vi "多道分析仪.vi"() -> ()   [LabVIEW 2014]
uses:
  <vilib>/Utility/miscctls.llb/LVPointDoubleTypeDef.ctl
  <vilib>/Utility/file.llb/Read From Spreadsheet File (DBL).vi
  <vilib>/Utility/file.llb/Write To Spreadsheet File (DBL).vi
  <vilib>/Analysis/NI_AAL_SigProc.lvlib
  <vilib>/Analysis/NI_AALPro.lvlib
panel:
  in  "按钮_对数":bool caption="对数"
  out "变量：显示数据":dbl[](array[numeric])
  out "状态：本次测量和上次未完成测量时间和":dbl
  out "状态：本次测试已测时间":dbl
  out "状态：上次未完成测试的已测时间":dbl
  out "变量：每次测量计划用时":u16=3600
  out "设置：幅度谱总道数 2":u32=4096
  out "变量：实时计数":i32
  out "变量：剩余使用时间":dbl
  out "center":dbl caption="中心"
  in  "设置：信号极性（正T）":bool=TRUE
  in  "数据缓存索引":u32
  out "变量 : 实时总计数":u64
  out "设置 ： 修正文件路径":path
  out "变量 ： 上次测量总计数":u32
  out "变量：上次测量原始数据":dbl[](array[numeric])
  out "状态：已测时间":dbl
  out "状态：测量开始时间":u32
  out "状态：刷新次数":i32
  in  "状态：停止变量":bool=TRUE
  out "变量：上次测量时间":dbl
  out "变量：原始数据":dbl[](array[numeric])
  out "MCA道宽修正数组":ext[](array[numeric])
  in  "设置：寻峰灵敏度":i32=3 caption="宽度" min=3
  in  "设置：甄别前阈值":u16=10000
  in  "设置：甄别后阈值":u16=9000
  in  "设置：刷新频率":u16
  in  "设置：测量时间":u16
  out "结果：净面积":dbl=1313865.0
  out "结果：半高宽":dbl=218.0
  out "结果：峰位":dbl=1585.0 caption="中心"
  in  "按钮_游标":bool caption="游标"
  in  "按钮_寻峰":T1 caption="寻峰"
  in  "按钮_右移":bool caption="右移"
  in  "按钮_还原":bool caption="还原"
  in  "按钮_放大":bool caption="放大"
  in  "按钮_左移":bool caption="左移"
  out "变量：感兴区终点道址":dbl=-1.0
  in  "显示：列表显示内容":string[](array[string])=["", "0秒", "正", "9000", "10000", "", "", "2014年3月7日", "0:56:44", "0秒", "0", "", "", "", "", "", "", "", "", "", "", ""]
  out "变量：感兴区起点道址":dbl=-1.0
  out "设置：幅度谱总道数":u32=4096
  in  "变量：图像缓存数组":dbl[][](array[numeric])
  in  "按钮_退出":bool caption="退出"
  in  "按钮_帮助":bool caption="帮助"
  in  "按钮_复位":bool caption="复位"
  in  "按钮_停止":bool caption="停止"
  in  "按钮_开始":bool caption="开始"
  in  "按钮_设置":bool caption="设置"
  in  "按钮_保存":bool caption="保存"
  in  "按钮_打开":bool caption="打开"
  out "显示：波形图":dbl[][](graph)
  out "显示：列表框":T2=6
  out "显示：波形图_预览":dbl[][](graph)
  out "状态栏_仪器状态":T3="核电子学硬件平台未连接" caption="状态栏"
  out "状态栏_剩余使用时间":T3="0" caption="剩余使用时间："
  out "状态栏_计数率":T3="0" caption="实时计数率："
  out "状态栏_游标状态":T3="隐藏" caption="游标状态："
  out "状态栏_游标计数":T3="0" caption="游标计数："
  out "状态栏_游标道址":T3="0" caption="游标道址："
  out "状态栏_测量状态":T3="停止" caption="测量状态："
  out "状态栏_日期":T3="2014/3/7   0:56:56" caption="日期"
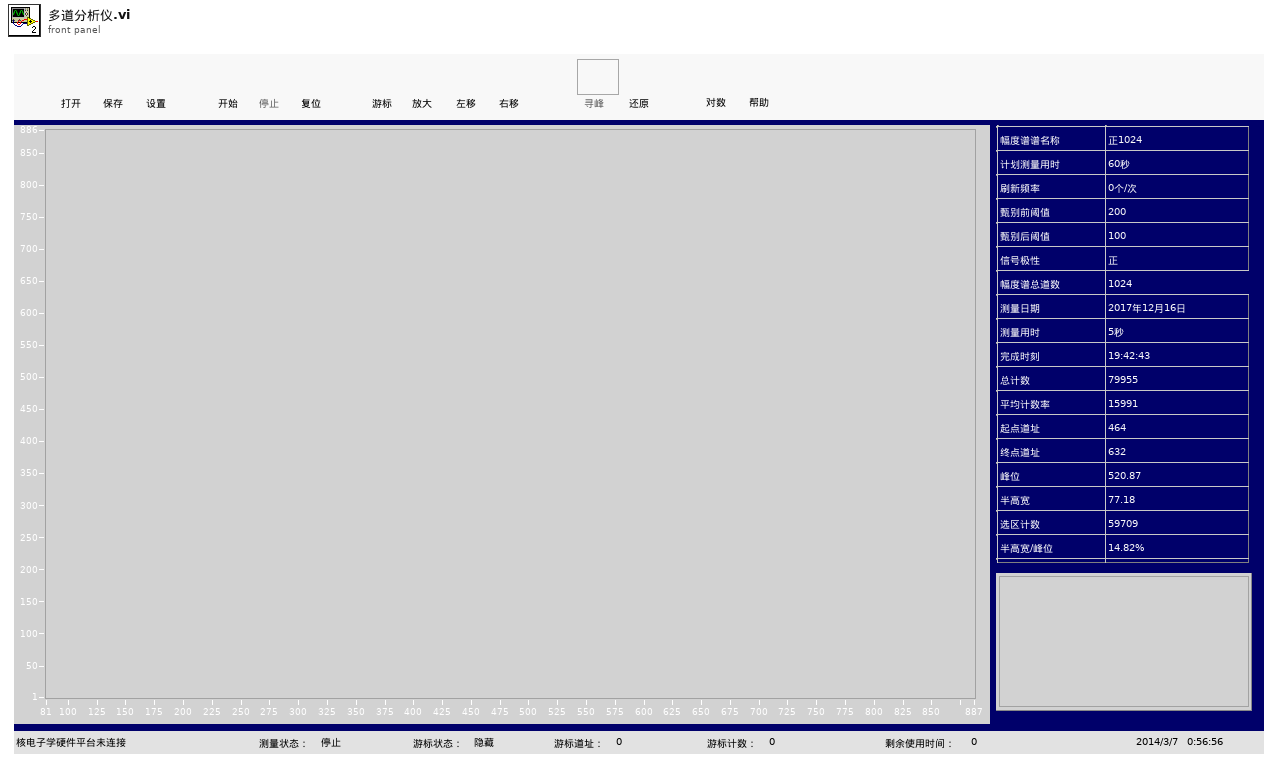
[diagram p1: front panel]
types:
  T1 = typedef "寻峰控件.ctl" = bool
  T2 = typedef "透明表格.ctl" = i32
  T3 = typedef "透明字符串.ctl" = string
  T4 = typedef "枚举常量_状态机.ctl" = enum16{"初始化", "等待", "完成"}
  T5 = typedef "LVPointDoubleTypeDef.ctl" = cluster{"X":dbl, "Y":dbl}
  T6 = enum8{"Enabled", "Disabled", "Disabled and Grayed Out"}
  T7 = enum16{"open", "open or create", "create or replace", "create", "open (read-only)"}
  T8 = typedef "eventvkey.ctl" = enum16{"ASCII", "Enter", "Return", "Shift", "Ctrl", "Alt", "Cmd", "Opt", "Caps", "NumLock", "Clear", "Break", "Up", "Down", "Left", "Right", "Insert", "Delete", "Home", "End", "PageUp", "PageDown", "Escape", "Help", "Pause", "ScrollLock", "F1", "F2", "F3", "F4", "F5", "F6", "F7", "F8", "F9", "F10", "F11", "F12", "F13", "F14", "F15", "F16", "F17", "F18", "F19", "F20", "F21", "F22", "F23", "F24", "Play", "VolumeUp", "VolumeDown", "Mute", "Two Byte Char"}
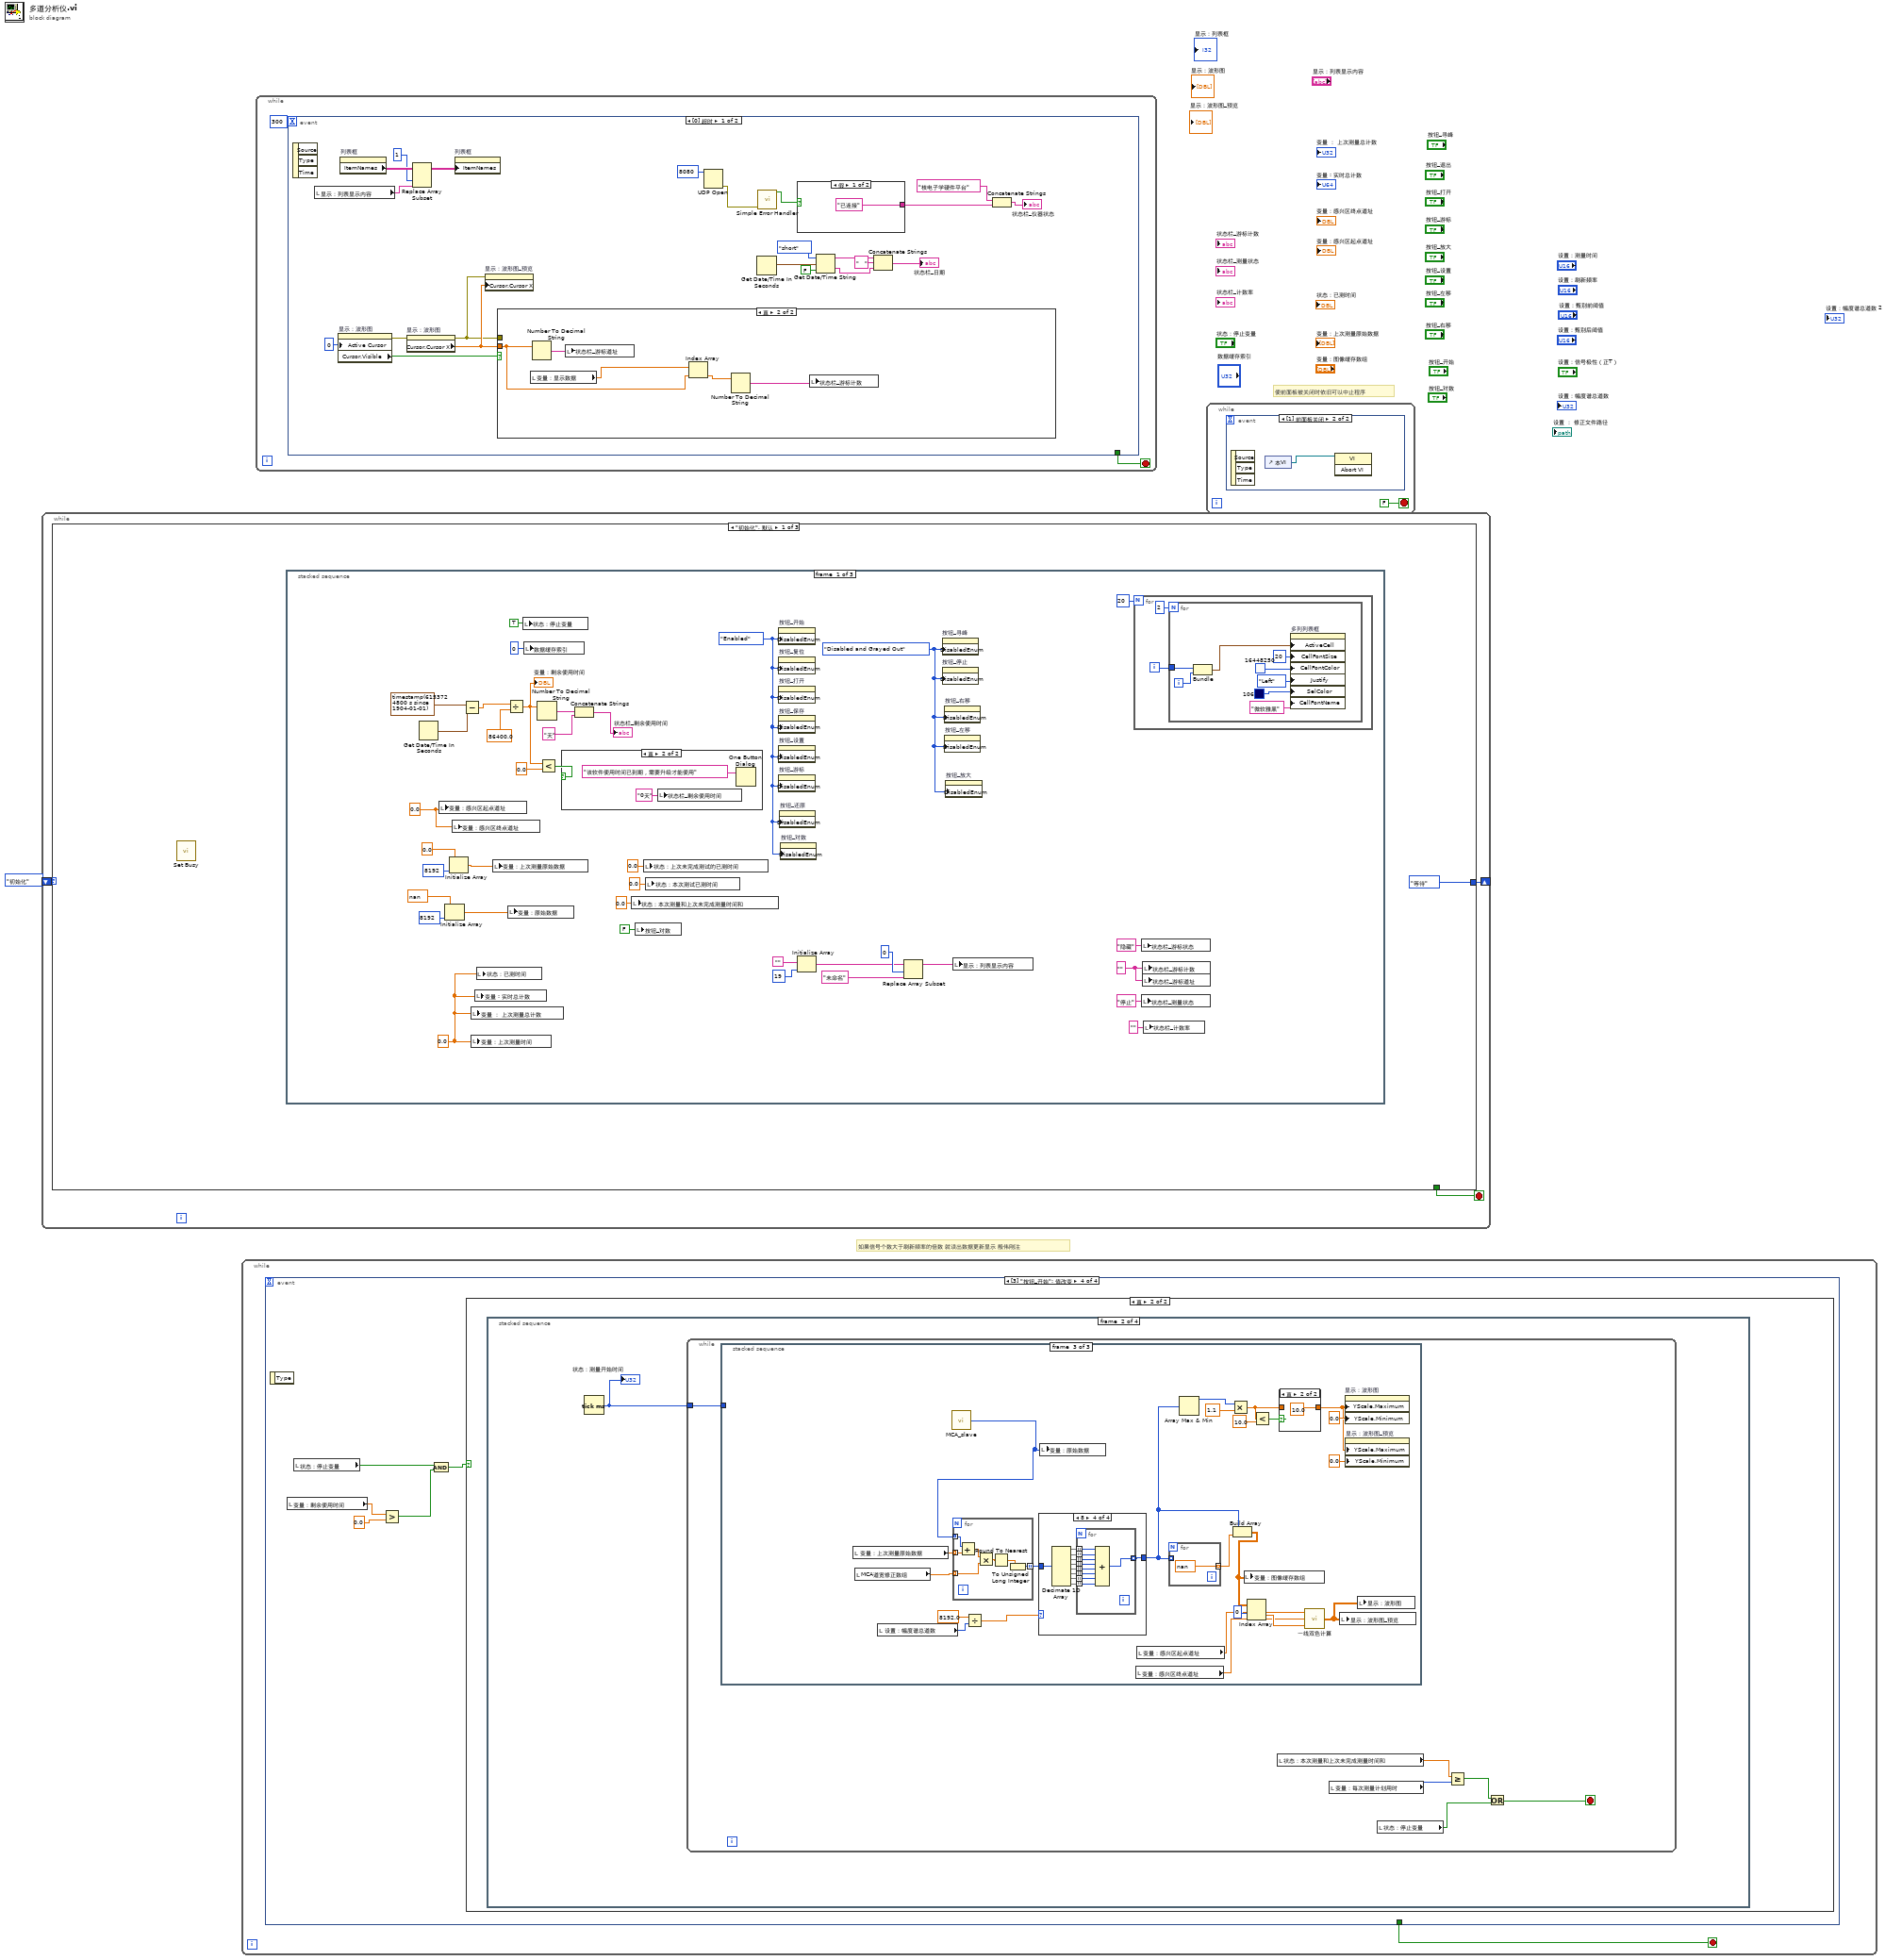
[diagram p0: block diagram]
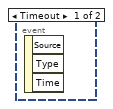
[diagram p2: hidden frame]
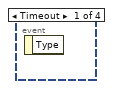
[diagram p3: hidden frame]
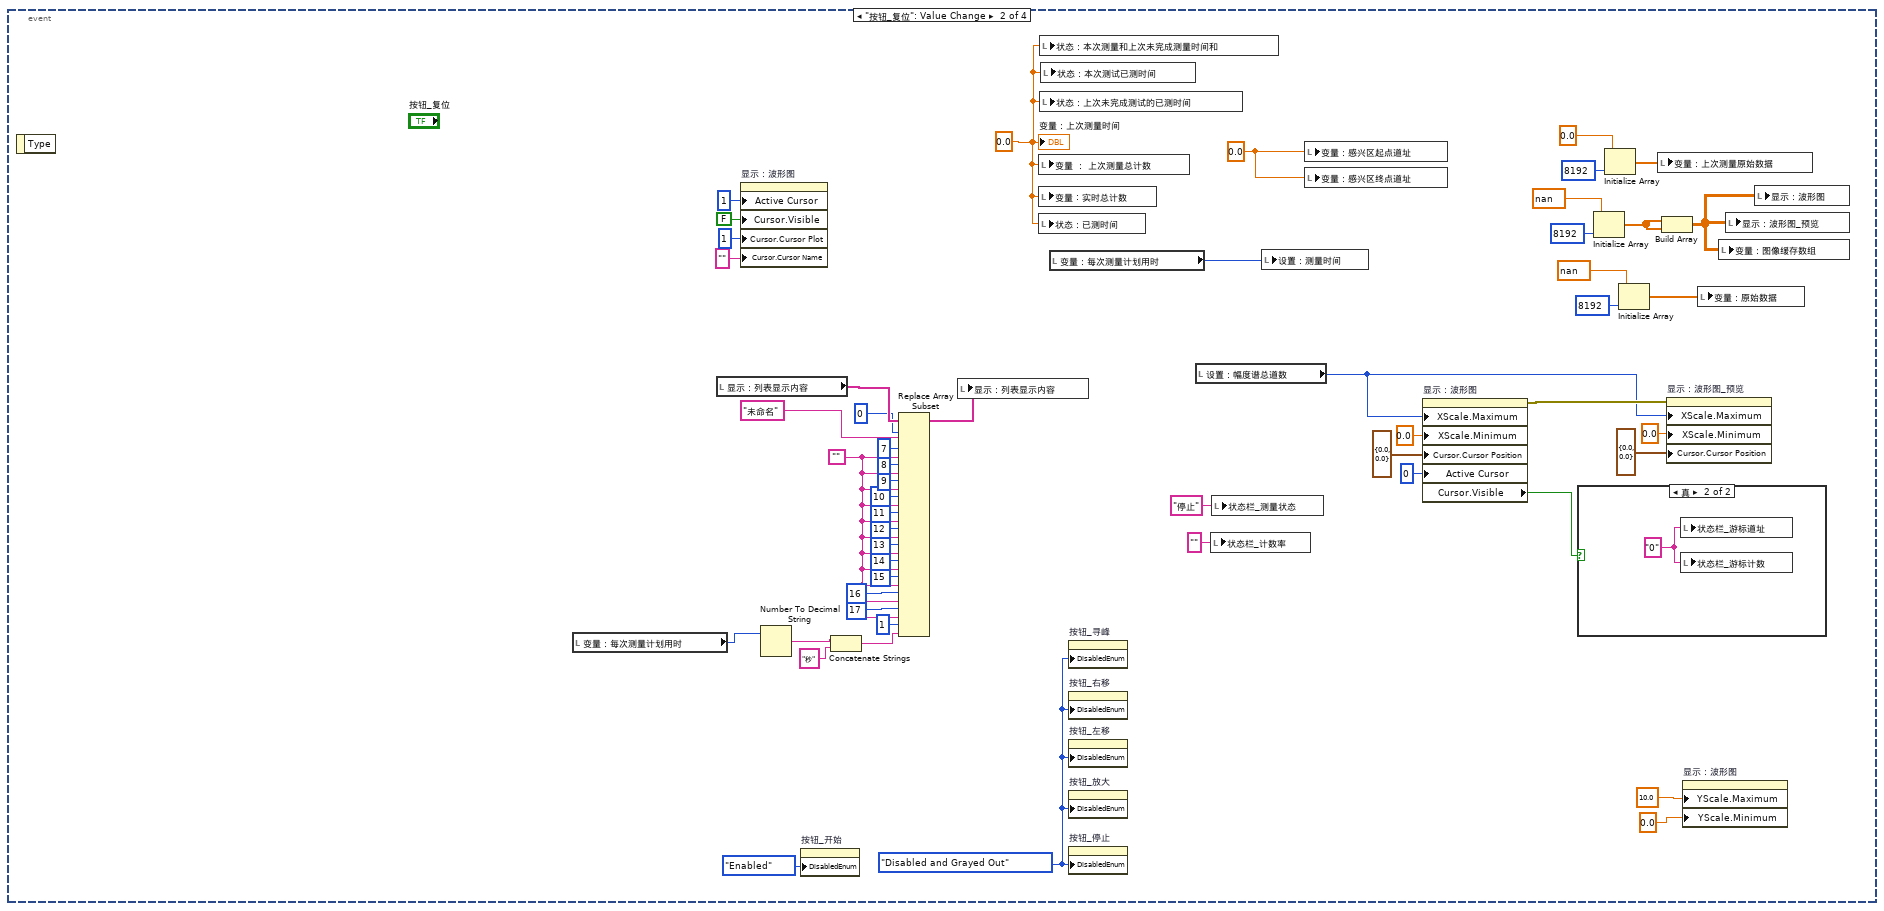
[diagram p4: hidden frame]
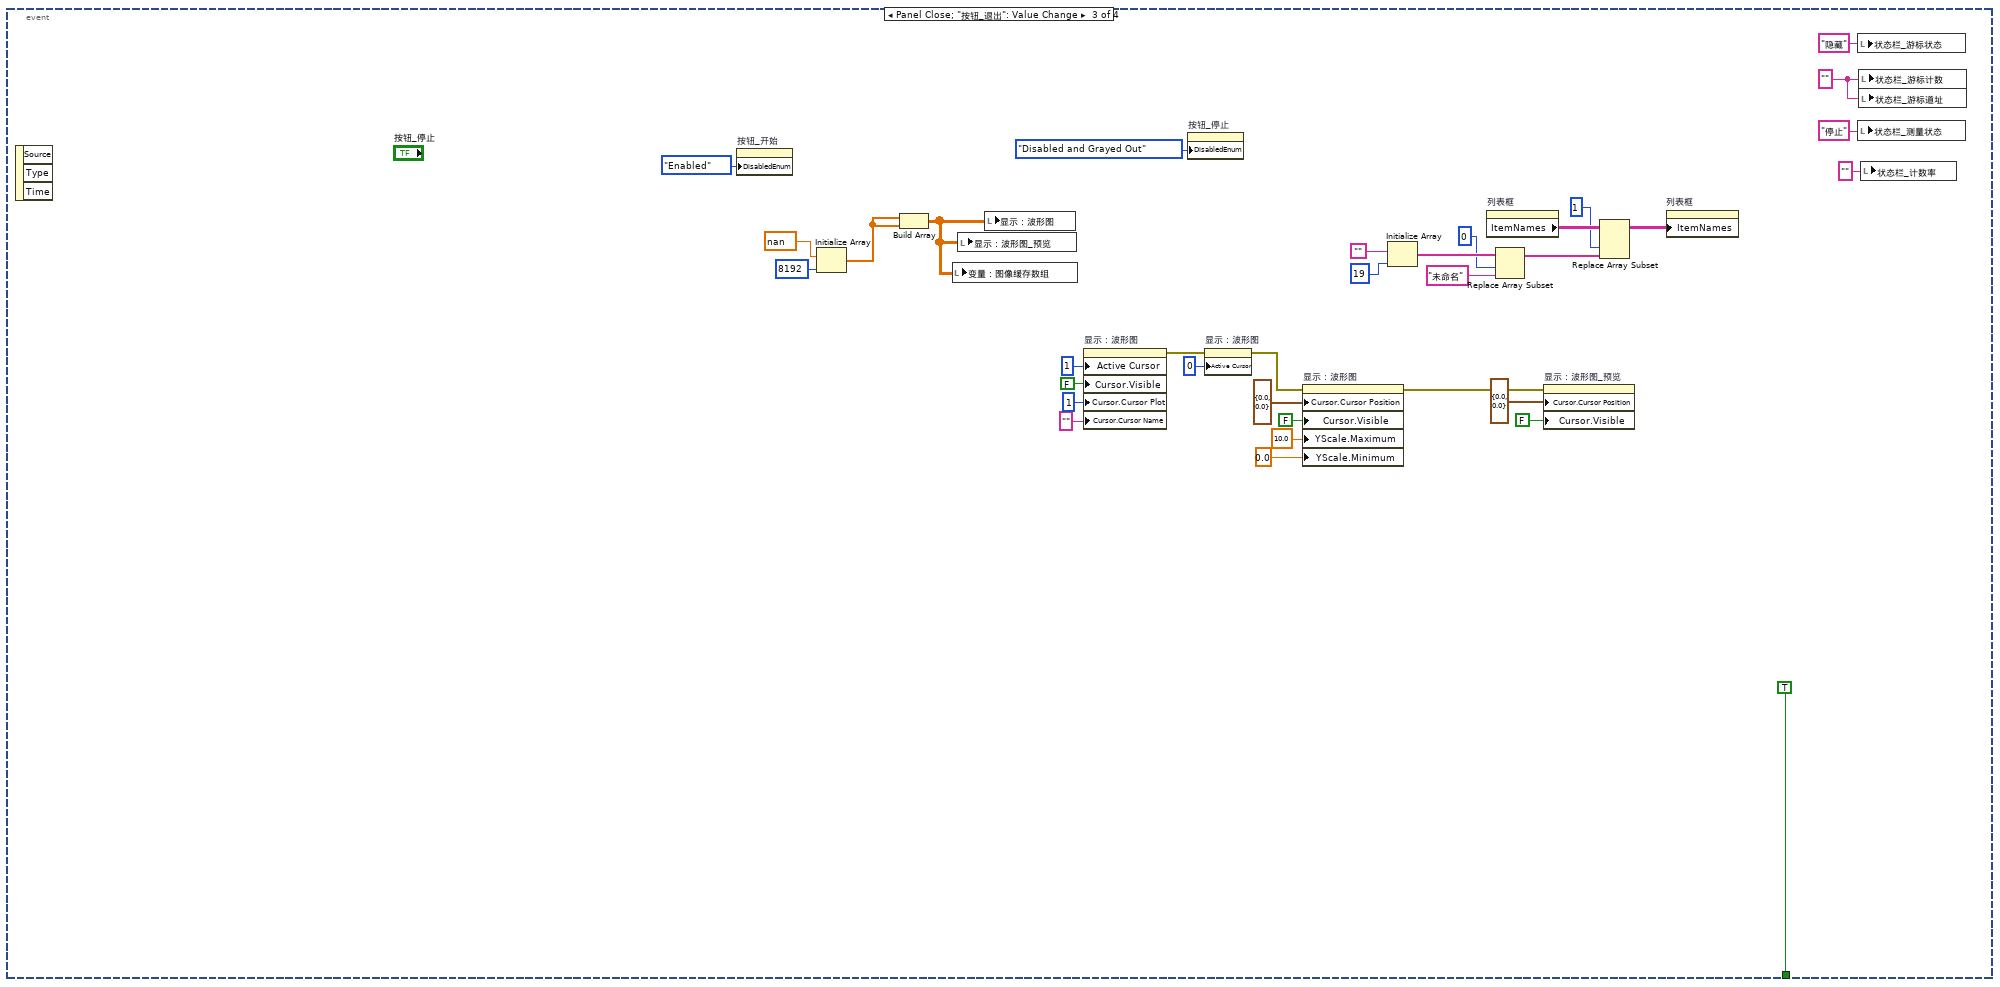
[diagram p6: hidden frame]
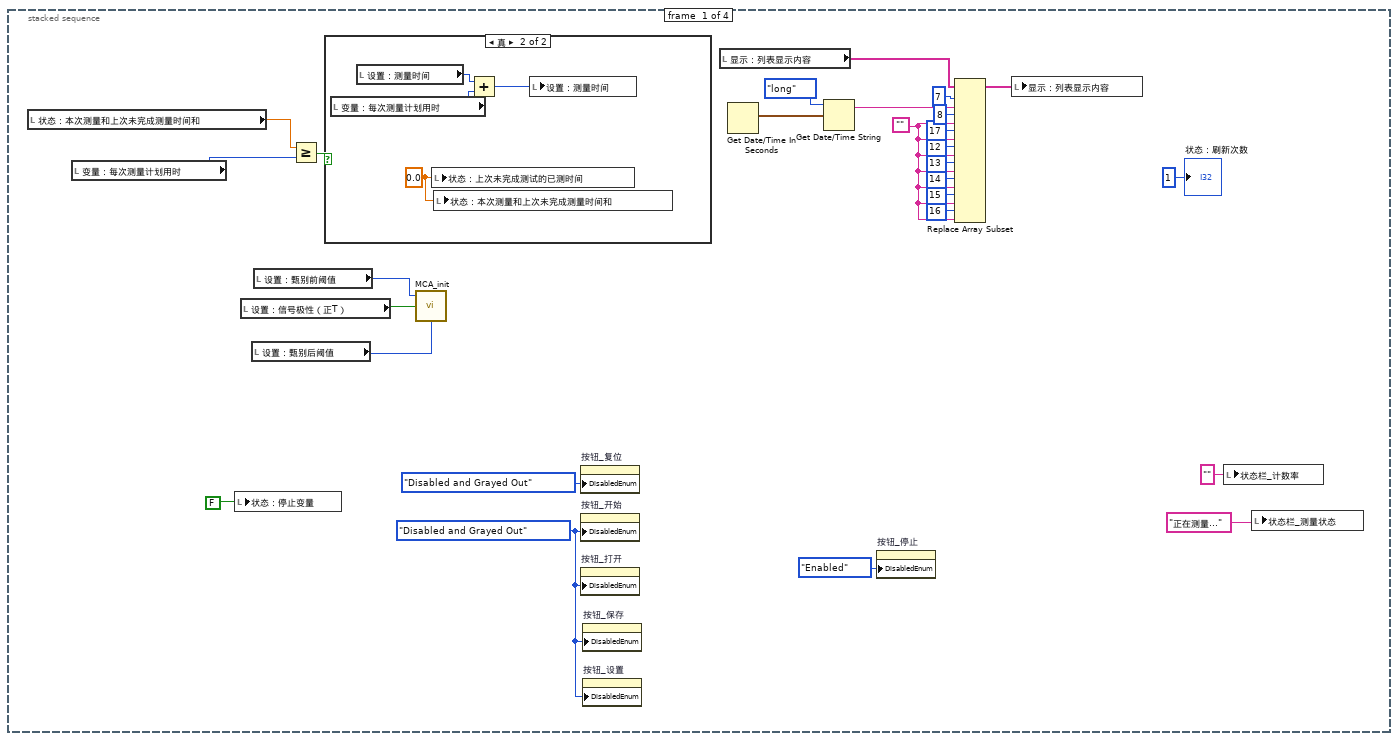
[diagram p8: hidden frame]
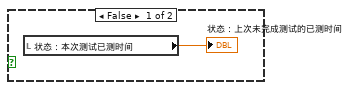
[diagram p9: hidden frame]
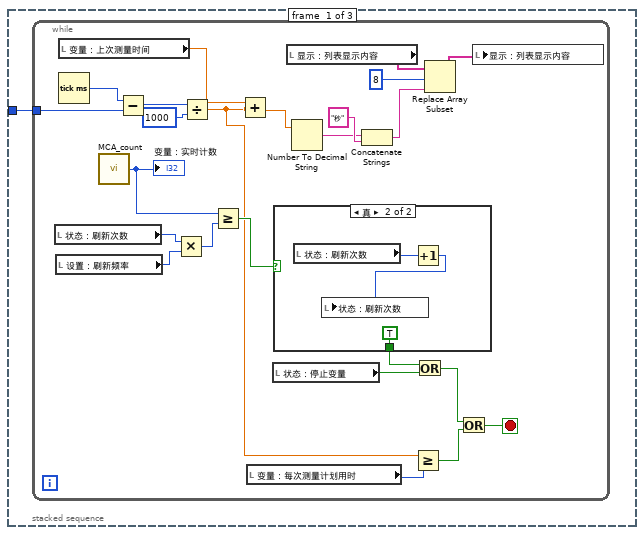
[diagram p10: hidden frame]
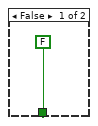
[diagram p11: hidden frame]
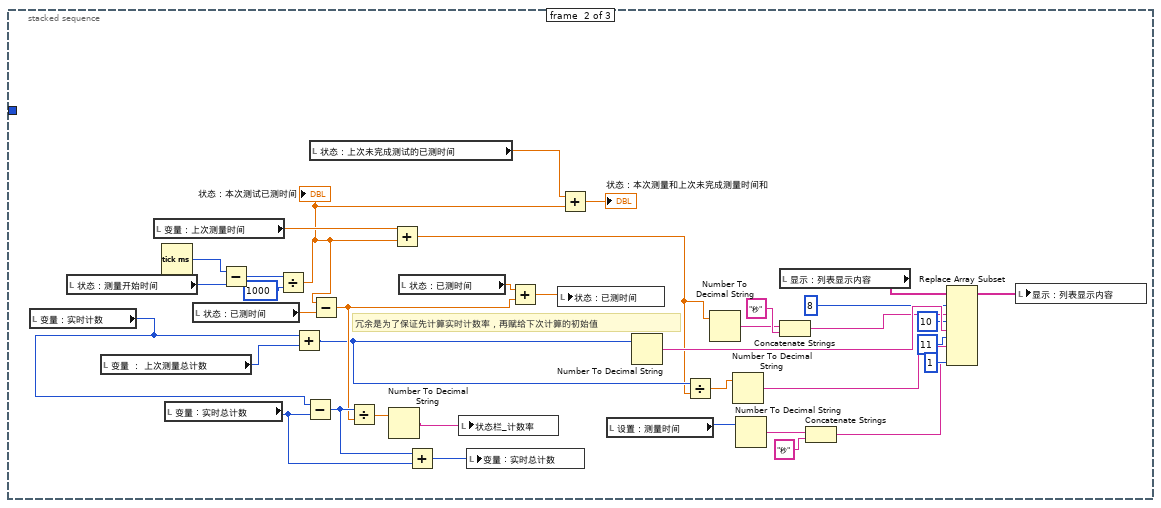
[diagram p12: hidden frame]
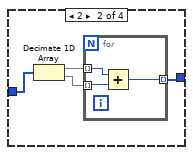
[diagram p15: hidden frame]
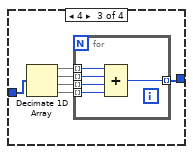
[diagram p16: hidden frame]
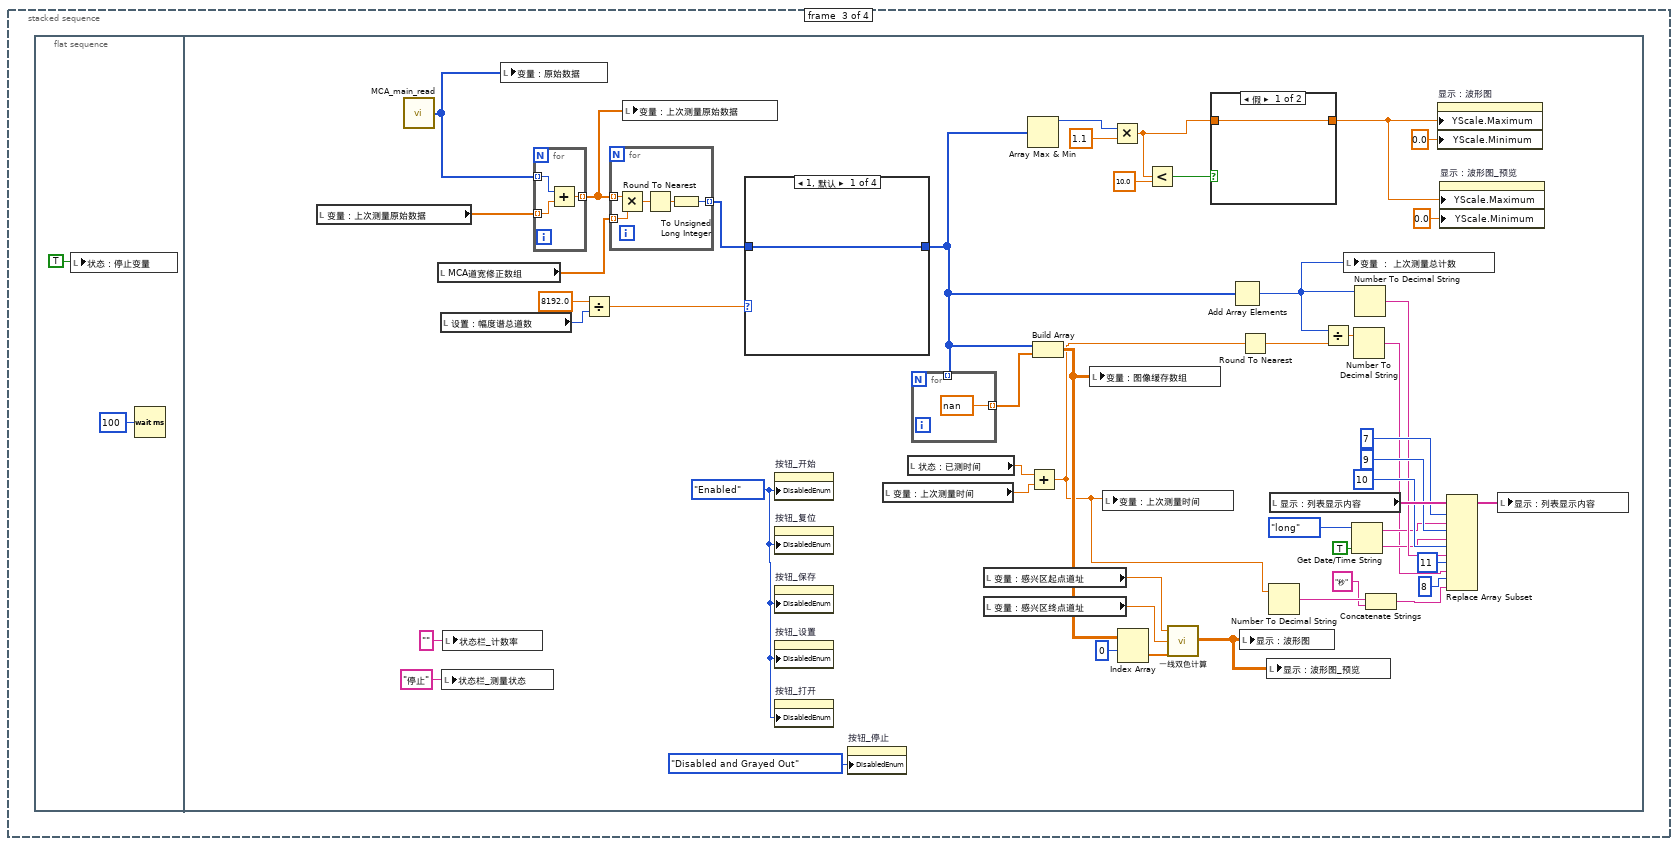
[diagram p17: hidden frame]
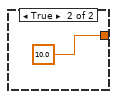
[diagram p18: hidden frame]
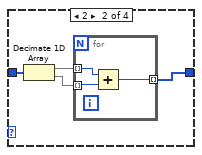
[diagram p19: hidden frame]
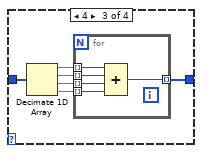
[diagram p20: hidden frame]
diagram:
  # "使前面板被关闭时依旧可以中止程序"
  # "如果信号个数大于刷新频率的倍数 就读出数据更新显示 殷伟刚注"
  n1 = while {
    shift-right: [w3] -> _
    shift-left: 枚举常量_状态机."初始化" ("枚举") -> [w4]
    stop <- w2 stop-if-true
    n2 = case shown="\"初始化\", 默认" w4 {
      tunnel: [枚举常量_状态机."等待" ("枚举") w124 枚举常量_状态机."完成" ("枚举")] -> w3
      tunnel: [_ _ TRUE] -> w2
      frame "初始化", Default {
        n3 = call <vilib>:"Set Busy.vi"() -> ()  [unwired: 10 in, 2 out]
        n4 = stacked-sequence {
          frame #0 {
            w30 = 0.0
            w27 = 0.0 ("变量：已测量时间")
            w7 = T6."Enabled" ("禁用")
            w39 = T3 "" ("状态栏_游标计数")
            w22 = T6."Disabled and Grayed Out" ("禁用")
            n5 = Get Date/Time In Seconds() -> (seconds since 1Jan1904=w14:timestamp)
            n6 = local write "变量：感兴区起点道址"(w30) -> ()
            n7 = Initialize Array(nan ("元素"), 8192 ("维数大小")) -> (w23:dbl[])
            n8 = Initialize Array(0.0 ("元素"), 8192 ("维数大小")) -> (w26:dbl[])
            n9 = local write "变量：感兴区终点道址"(w30) -> ()
            n10 = Subtract(x=timestamp(6153724800 s since 1904-01-01), y=w14) -> (x-y=w16:dbl)
            n11 = local write "变量 ： 上次测量总计数"(w27) -> ()
            n12 = local write "变量：上次测量时间"(w27) -> ()
            n13 = local write "变量 : 实时总计数"(w27) -> ()
            n14 = local write "状态：已测时间"(w27) -> ()
            n15 = local write "变量：上次测量原始数据"(w26) -> ()
            n16 = Divide(x=w16, y=86400.0) -> (x/y=w13:dbl)
            "变量：剩余使用时间" <- w13
            n17 = local write "变量：原始数据"(w23) -> ()
            n18 = local write "状态：停止变量"(TRUE ("停止变量")) -> ()
            n19 = local write "数据缓存索引"(u32 0 ("数据缓存索引")) -> ()
            n20 = Number To Decimal String(number=w13) -> (decimal integer string=w18:string)  [unwired: 1 in]
            n21 = Less?(x=w13, y=0.0) -> (x < y?=w11:bool)
            n22 = case shown="真" w11 {
              frame False {
              }
              frame True {
                n23 = local write "状态栏_剩余使用时间"(T3 "0天" ("状态栏_剩余使用时间")) -> ()
                n24 = One Button Dialog(message="该软件使用时间已到期，需要升级才能使用" ("消息")) -> ()  [unwired: 1 in, 1 out]
              }
            }
            n25 = Concatenate Strings(w18, "天" ("字符串")) -> (→"状态栏_剩余使用时间":string)
            n26 = local write "状态：本次测量和上次未完成测量时间和"(0.0 ("状态：本次测量和上次未完成测量时间和")) -> ()
            n27 = local write "按钮_对数"(FALSE ("按钮_对数")) -> ()
            n28 = local write "状态：上次未完成测试的已测时间"(0.0 ("状态：上次未完成测试的已测时间")) -> ()
            n29 = local write "状态：本次测试已测时间"(0.0 ("状态：本次测试已测时间")) -> ()
            n30 = property on="按钮_开始" class="Bool"("DisabledEnum"=w7) -> ()  [unwired: 2 in, 2 out]
            n31 = property on="按钮_复位" class="Bool"("DisabledEnum"=w7) -> ()  [unwired: 2 in, 2 out]
            n32 = property on="按钮_打开" class="Bool"("DisabledEnum"=w7) -> ()  [unwired: 2 in, 2 out]
            n33 = property on="按钮_保存" class="Bool"("DisabledEnum"=w7) -> ()  [unwired: 2 in, 2 out]
            n34 = property on="按钮_设置" class="Bool"("DisabledEnum"=w7) -> ()  [unwired: 2 in, 2 out]
            n35 = property on="按钮_游标" class="Bool"("DisabledEnum"=w7) -> ()  [unwired: 2 in, 2 out]
            n36 = property on="按钮_还原" class="Bool"("DisabledEnum"=w7) -> ()  [unwired: 2 in, 2 out]
            n37 = property on="按钮_对数" class="Bool (严格)"("DisabledEnum"=w7) -> ()  [unwired: 2 in, 2 out]
            n38 = Initialize Array("", 19 ("维数大小")) -> (w32:string[])
            n39 = Replace Array Subset(array=w32, new element="未命名" ("新元素/子数组"), index=0 ("索引")) -> (w37:string[])
            n40 = property on="按钮_寻峰" class="Bool"("DisabledEnum"=w22) -> ()  [unwired: 2 in, 2 out]
            n41 = property on="按钮_停止" class="Bool (严格)"("DisabledEnum"=w22) -> ()  [unwired: 2 in, 2 out]
            n42 = property on="按钮_右移" class="Bool"("DisabledEnum"=w22) -> ()  [unwired: 2 in, 2 out]
            n43 = property on="按钮_左移" class="Bool"("DisabledEnum"=w22) -> ()  [unwired: 2 in, 2 out]
            n44 = property on="按钮_放大" class="Bool"("DisabledEnum"=w22) -> ()  [unwired: 2 in, 2 out]
            n45 = local write "显示：列表显示内容"(w37) -> ()
            n46 = for {
              N: 20 -> [_]
              i -> [w45]
              n47 = for {
                N: 2 -> [_]
                tunnel: w45 -> [w53]
                i -> [w54]
                n48 = Bundle(w53, w54) -> (w52:cluster{i32, i32})  [unwired: 1 in]
                n49 = property on="多列列表框" class="MCListbox (严格)"("ActiveCell"=w52, "CellFontSize"=u32 20 ("活动单元格:单元格字体:字号"), "CellFontColor"=u32 16448250 ("Color"), "Justify"=enum16{"Left", "Center", "Right"}."Left" ("活动单元格:单元格对齐"), "SelColor"=u32 106 ("Color"), "CellFontName"="微软雅黑" ("活动单元格:单元格字体:名称")) -> ()  [unwired: 2 in, 2 out]
              }
            }
            n50 = local write "状态栏_游标状态"(T3 "隐藏" ("状态栏_游标状态")) -> ()
            n51 = local write "状态栏_测量状态"(T3 "停止" ("状态栏_测量状态")) -> ()
            n52 = local write "状态栏_游标计数"(w39) -> ()
            n53 = local write "状态栏_游标道址"(w39) -> ()
            n54 = local write "状态栏_计数率"(T3 "" ("状态栏_计数率")) -> ()
          }
          frame #1 {
            # "此处得到MCA道宽不均匀修正数组"
            n55 = call "MCA_ReadConfig.vi"() -> ("数据刷新频率"=w60:u16, "测量最多花费的时间（秒）："=w61:u16, "甄别后阈值"=w62:u16, "甄别前阈值"=w63:u16, "寻峰灵敏度"=w59:u16, "最大道数"=w57:u16, "数据文件路径"=w58:path, "信号极性"=w64:bool)  [unwired: 3 in, 1 out]
            "变量：每次测量计划用时" <- w61
            n56 = local write "设置：信号极性（正T）"(w64) -> ()
            n57 = local write "设置：幅度谱总道数"(w57) -> ()
            n58 = local write "设置：甄别前阈值"(w63) -> ()
            n59 = local write "设置：甄别后阈值"(w62) -> ()
            n60 = local write "设置：测量时间"(w61) -> ()
            n61 = local write "设置：刷新频率"(w60) -> ()
            n62 = local write "设置：寻峰灵敏度"(w59) -> ()
            n63 = Equal?(x=w58, y=path "") -> (x = y?=w86:bool)
            n64 = case shown="真" w86 {
              tunnel: w58 -> [w91 _]
              tunnel: [w89 w92] -> w65
              frame False {
                n65 = call-poly <vilib>:"Read From Spreadsheet File.vi"("transpose (no:F)"=TRUE, "file path (dialog if empty)"=w91) -> ("first row"=w89:dbl[])  [unwired: 5 in, 4 out]
              }
              frame True {
                n66 = Initialize Array(1.0 ("元素"), 8192 ("维数大小")) -> (w92:dbl[])
              }
            }
            "MCA道宽修正数组" <- w65
            n67 = local write "设置 ： 修正文件路径"(w58) -> ()
            n68 = property on="显示：波形图" class="WFGraph (严格)"("Active Cursor"=u32 1 ("活动游标"), "Cursor.Visible"=FALSE ("游标.可见"), "Cursor.Cursor Plot"=1 ("游标.游标关联曲线"), "Cursor.Cursor Name"="" ("游标.游标名")) -> (error out=w69:errorcluster)  [unwired: 2 in, 1 out]
            n69 = property on="显示：波形图" class="WFGraph (严格)"(error in=w69, "Active Cursor"=u32 0 ("活动游标")) -> (error out=w74:errorcluster)  [unwired: 1 in, 1 out]
            n70 = property on="显示：波形图" class="WFGraph (严格)"(error in=w74, "XScale.Maximum"=w57, "XScale.Minimum"=0.0 ("X标尺.范围:最小值"), "Cursor.Cursor Position"=T5 {"X"=0.0, "Y"=0.0} ("游标.游标位置"), "Cursor.Visible"=FALSE ("游标.可见"), "YScale.Maximum"=10.0 ("Y标尺.范围:最大值"), "YScale.Minimum"=0.0 ("Y标尺.范围:最小值"), "YScale.Mapping Mode"=u8 0 ("Y标尺.映射模式")) -> (error out=w77:errorcluster)  [unwired: 1 in, 1 out]
            n71 = Initialize Array(nan ("元素"), w57) -> (w85:dbl[])
            n72 = for {
              tunnel: w85 -> [_] mode=indexing
              tunnel: [nan] -> w82 mode=indexing
            }
            n73 = property on="显示：波形图_预览" class="WFGraph (严格)"(error in=w77, "XScale.Maximum"=w57, "XScale.Minimum"=0.0 ("X标尺.范围:最小值"), "Cursor.Cursor Position"=T5 {"X"=0.0, "Y"=0.0} ("游标.游标位置"), "Cursor.Visible"=FALSE ("游标.可见"), "YScale.Mapping Mode"=u8 0 ("Y标尺.映射模式")) -> ()  [unwired: 1 in, 2 out]
            n74 = Build Array(w85, w82) -> (w83:dbl[][])
            n75 = local write "显示：波形图_预览"(w83) -> ()
            n76 = local write "变量：图像缓存数组"(w83) -> ()
            n77 = local write "显示：波形图"(w83) -> ()
          }
          frame #2 {
            n78 = local read "设置：信号极性（正T）"() -> (w102:bool)
            n79 = local read "设置：寻峰灵敏度"() -> (w105:i32)
            n80 = local read "设置：幅度谱总道数"() -> (w97:u32)
            n81 = local read "设置：测量时间"() -> (w109:u16)
            n82 = local read "设置：刷新频率"() -> (w108:u16)
            n83 = local read "设置：甄别后阈值"() -> (w106:u16)
            n84 = local read "设置：甄别前阈值"() -> (w107:u16)
            n85 = case shown="假" w102 {
              tunnel: ["负" ("字符串") "正" ("字符串")] -> w101
              frame False {
              }
              frame True {
              }
            }
            n86 = Number To Decimal String(number=w105) -> (decimal integer string=w99:string)  [unwired: 1 in]
            n87 = Number To Decimal String(number=w97) -> (decimal integer string=w96:string)  [unwired: 1 in]
            n88 = Number To Decimal String(number=w109) -> (decimal integer string=w114:string)  [unwired: 1 in]
            n89 = Number To Decimal String(number=w106) -> (decimal integer string=w103:string)  [unwired: 1 in]
            n90 = Number To Decimal String(number=w108) -> (decimal integer string=w119:string)  [unwired: 1 in]
            n91 = Number To Decimal String(number=w107) -> (decimal integer string=w104:string)  [unwired: 1 in]
            n92 = Concatenate Strings(w114, "秒" ("字符串")) -> (w115:string)
            n93 = Concatenate Strings(w119, "个/次" ("字符串")) -> (w121:string)
            n94 = local read "显示：列表显示内容"() -> (w111:string[])
            n95 = Replace Array Subset(array=w111, new element #1=w115, index #1=1 ("索引"), new element #2=w121, index #2=2 ("索引"), new element #3=w104, index #3=3 ("索引"), new element #4=w103, index #4=4 ("索引"), new element #5=w101, index #5=5 ("索引"), new element #6=w96, index #6=6 ("索引"), new element #7=w99, index #7=18 ("索引")) -> (w112:string[])
            n96 = local write "显示：列表显示内容"(w112) -> ()
          }
        }
      }
      frame "等待" {
        n97 = call <vilib>:"Unset Busy.vi"() -> ()  [unwired: 11 in, 1 out]
        n98 = event shown="[8] \"按钮_对数\": 值改变" {
          selector: _ -> [_ _ _ _ _ _ _ _ _ _ _ _ _ _ _ _ _ _]
          dyn-events: _ -> [_ _ _ _ _ _ _ _ _ _ _ _ _ _ _ _ _ _]
          timeout: _ -> [_ _ _ _ _ _ _ _ _ _ _ _ _ _ _ _ _ _]
          tunnel: [枚举常量_状态机."等待" ("枚举") 枚举常量_状态机."等待" ("枚举") 枚举常量_状态机."完成" ("枚举") 枚举常量_状态机."等待" ("枚举") 枚举常量_状态机."等待" ("枚举") 枚举常量_状态机."等待" ("枚举") 枚举常量_状态机."等待" ("枚举") 枚举常量_状态机."等待" ("枚举") 枚举常量_状态机."等待" ("枚举") 枚举常量_状态机."等待" ("枚举") 枚举常量_状态机."等待" ("枚举") 枚举常量_状态机."等待" ("枚举") 枚举常量_状态机."等待" ("枚举") 枚举常量_状态机."等待" ("枚举") 枚举常量_状态机."等待" ("枚举") 枚举常量_状态机."等待" ("枚举") 枚举常量_状态机."等待" ("枚举") 枚举常量_状态机."等待" ("枚举")] -> w124
          event Timeout {
            n99 = event-data() -> ()  [unwired: 1 in, 3 out]
          }
          event "按钮_帮助": Value Change {
            n100 = event-data() -> ()  [unwired: 1 in, 6 out]
            n101 = call "显示对话框信息"() -> ("软件介绍"=w126:bool)  [unwired: 10 in, 1 out]
            n102 = case shown="真" w126 {
              frame False {
              }
              frame True {
                n103 = call "显示对话框信息2"() -> ()  [unwired: 10 in, 2 out]
              }
            }
          }
          event "按钮_退出": Value Change {
            n104 = event-data() -> ()  [unwired: 1 in, 6 out]
            n105 = local write "状态：停止变量"(TRUE ("停止变量")) -> ()
          }
          event "按钮_停止": Value Change {
            w133 = T6."Enabled" ("禁用")
            n106 = event-data() -> ()  [unwired: 1 in, 6 out]
            n107 = property on="按钮_复位" class="Bool"("DisabledEnum"=w133) -> ()  [unwired: 2 in, 2 out]
            n108 = property on="按钮_开始" class="Bool"("DisabledEnum"=T6."Enabled" ("禁用")) -> ()  [unwired: 2 in, 2 out]
            n109 = property on="按钮_打开" class="Bool"("DisabledEnum"=w133) -> ()  [unwired: 2 in, 2 out]
            n110 = property on="按钮_保存" class="Bool"("DisabledEnum"=w133) -> ()  [unwired: 2 in, 2 out]
            n111 = property on="按钮_设置" class="Bool"("DisabledEnum"=w133) -> ()  [unwired: 2 in, 2 out]
            n112 = local write "状态：停止变量"(TRUE ("停止变量")) -> ()
            n113 = property on="按钮_停止" class="Bool (严格)"("Value"=FALSE ("停止"), "DisabledEnum"=T6."Disabled and Grayed Out" ("禁用")) -> ()  [unwired: 2 in, 2 out]
          }
          event "显示：波形图": Cursor Move {
            n114 = event-data() -> ()  [unwired: 1 in, 9 out]
            n115 = property on="显示：波形图" class="WFGraph (严格)"() -> ("Cursor.Cursor Position"=w143:T5)  [unwired: 2 in, 2 out]
            n116 = property on="显示：波形图_预览" class="WFGraph (严格)"("Cursor.Cursor Position"=w143) -> ()  [unwired: 2 in, 2 out]
            n117 = Unbundle By Name(w143) -> ("Cursor X"=w140:dbl, "Cursor Y"=w139:dbl)
            n118 = Number To Decimal String(number=w140) -> (decimal integer string=→"状态栏_游标道址":string)  [unwired: 1 in]
            n119 = Number To Decimal String(number=w139) -> (decimal integer string=w138:string)  [unwired: 1 in]
            n120 = Equal?(x=w138, y="NaN") -> (x = y?=w144:bool)
            n121 = case shown="真" w144 {
              tunnel: [w146 w152] -> w141
              tunnel: w139 -> [w146 _]
              frame False {
              }
              frame True {
                n122 = property on="显示：波形图" class="WFGraph (严格)"() -> (error out=w153:errorcluster, "Cursor.Cursor Plot"=w149:i32)  [unwired: 2 in, 1 out]
                n123 = Equal To 0?(x=w149) -> (x = 0?=w150:bool)
                n124 = Select(t=1.0, s=w150, f=0.0) -> (s? t:f=w151:dbl)
                n125 = property on="显示：波形图" class="WFGraph (严格)"(error in=w153, "Cursor.Cursor Plot"=w151) -> ("Cursor.Cursor Y"=w152:dbl)  [unwired: 1 in, 2 out]
              }
            }
            n126 = Number To Decimal String(number=w141) -> (decimal integer string=w136:string)  [unwired: 1 in]
            n127 = local write "状态栏_游标计数"(w136) -> ()
          }
          event "按钮_打开": Value Change {
            n128 = event-data() -> ()  [unwired: 1 in, 1 out]
            n129 = call "MCA_OpenDialog.vi"() -> ("要打开的数据文件路径： 2"=w154:path, "是否取消？"=w155:bool)  [unwired: 10 in]
            n130 = case shown="假" w155 {
              tunnel: w154 -> [w157 _]
              frame False {
                n131 = Strip Path(path=w157) -> (name=w164:string)  [unwired: 1 out]
                n132 = String Length(string=w164) -> (length=w163:i32)
                n133 = Subtract(x=w163, y=4) -> (x-y=w161:i32)
                n134 = String Subset(string=w164, offset (0)=w161, length (rest)=w163) -> (substring=w160:string)
                n135 = Equal?(x=w160, y="tdms") -> (x = y?=w158:bool)
                n136 = case shown="真" w158 {
                  tunnel: w157 -> [w166 w198]
                  frame False {
                    n137 = Strip Path(path=w166) -> (name=w165:string)  [unwired: 1 out]
                    n138 = String Length(string=w165) -> (length=w172:i32)
                    n139 = Subtract(x=w172, y=4) -> (x-y=w170:i32)
                    n140 = String Subset(string=w165, offset (0)=w170, length (rest)=w172) -> (substring=w169:string)
                    n141 = Equal?(x=w169, y=".txt") -> (x = y?=w167:bool)
                    n142 = case shown="真" w167 {
                      tunnel: w166 -> [_ w174]
                      tunnel: w165 -> [_ w173]
                      frame False {
                      }
                      frame True {
                        n143 = flat-sequence {
                          tunnel: w174 -> [w189]
                          tunnel: w173 -> [w178]
                          frame #0 {
                            n144 = call-poly <vilib>:"Read From Spreadsheet File.vi"("transpose (no:F)"=TRUE, "file path (dialog if empty)"=w189) -> ("first row"=w175:dbl[])  [unwired: 5 in, 4 out]
                            n145 = local read "显示：列表显示内容"() -> (w179:string[])
                            n146 = local read "设置：幅度谱总道数"() -> (w184:u32)
                            n147 = Replace Array Subset(array=w179, new element=w178, index=0 ("索引")) -> (w176:string[])
                            n148 = local write "显示：列表显示内容"(w176) -> ()
                            n149 = local write "变量：原始数据"(w175) -> ()
                            n150 = Array Max & Min(array=w175) -> (max value=w183:dbl)  [unwired: 3 out]
                            n151 = Initialize Array(nan ("元素"), w184) -> (w187:dbl[])
                            n152 = Build Array(w175, w187) -> (w188:dbl[][])
                            n153 = Multiply(x=w183, y=1.1) -> (x*y=w181:dbl)
                            n154 = local write "显示：波形图"(w188) -> ()
                            n155 = local write "显示：波形图_预览"(w188) -> ()
                            n156 = local write "变量：图像缓存数组"(w188) -> ()
                            n157 = property on="显示：波形图" class="WFGraph (严格)"("YScale.Maximum"=w181, "YScale.Minimum"=0.0 ("Y标尺.范围:最小值")) -> ()  [unwired: 2 in, 2 out]
                            n158 = property on="显示：波形图_预览" class="WFGraph (严格)"("YScale.Maximum"=w181, "YScale.Minimum"=0.0 ("Y标尺.范围:最小值")) -> ()  [unwired: 2 in, 2 out]
                          }
                          frame #1 {
                            w196 = T5 {"X"=0.0, "Y"=0.0} ("游标.游标位置")
                            n159 = local read "设置：幅度谱总道数"() -> (w197:u32)
                            n160 = property on="显示：波形图_预览" class="WFGraph (严格)"("Cursor.Cursor Position"=w196, "XScale.Maximum"=w197, "XScale.Minimum"=0.0 ("X标尺.范围:最小值")) -> ()  [unwired: 2 in, 2 out]
                            n161 = property on="显示：波形图" class="WFGraph (严格)"("XScale.Maximum"=w197, "XScale.Minimum"=0.0 ("X标尺.范围:最小值"), "Cursor.Cursor Position"=w196, "ActPaletteTool"=0 ("选板:活动工具"), "Plot.Visible?"=TRUE ("曲线.可见"), "Active Plot"=u32 1 ("活动曲线")) -> ()  [unwired: 2 in, 2 out]
                          }
                        }
                      }
                    }
                  }
                  frame True {
                    n162 = flat-sequence {
                      tunnel: w198 -> [w201]
                      frame #0 {
                        n163 = TDMS Open(5:FALSE ("创建索引文件？(T)"), 10:T7."open" ("操作(0:open)"), 11:w201) -> (0:w208:errorcluster, 3:w218:refnum<k34>)  [unwired: 4 in]
                        n164 = TDMS Read(0:w218, 5:"文件属性" ("组名称输入"), 11:w208, 12:string[][] []) -> (4:w212:refnum<k34>, 10:w216:string[][], 15:w207:errorcluster)  [unwired: 4 in, 3 out]
                        n165 = Index Array(array=w216, index (row)=1 ("索引")) -> (element=w214:string[])  [unwired: 1 in]
                        n166 = local write "显示：列表显示内容"(w214) -> ()
                        n167 = TDMS Read(0:w212, 5:"数据" ("组名称输入"), 11:w207, 12:dbl[] []) -> (4:w209:refnum<k34>, 10:w200:dbl[], 15:w206:errorcluster)  [unwired: 4 in, 3 out]
                        "变量：原始数据" <- w200
                        n168 = local read "设置：幅度谱总道数"() -> (w205:u32)
                        n169 = TDMS Close(8:w206, 11:w209) -> ()  [unwired: 2 out]
                        n170 = case shown="1024, 默认" w205 {
                          tunnel: w200 -> [w226 w230 w234 w254]
                          tunnel: [w226 w227 w237 w251] -> w199
                          frame 8192 {
                          }
                          frame 4096 {
                            n171 = Decimate 1D Array(w230) -> (w228:dbl[], w229:dbl[])
                            n172 = for {
                              tunnel: w229 -> [w232] mode=indexing
                              tunnel: w228 -> [w233] mode=indexing
                              tunnel: [w231] -> w227 mode=indexing
                              n173 = Add(x=w233, y=w232) -> (x+y=w231:dbl)
                            }
                          }
                          frame 2048 {
                            n174 = Decimate 1D Array(w234) -> (w238:dbl[], w239:dbl[], w236:dbl[], w235:dbl[])
                            n175 = for {
                              tunnel: w239 -> [w243] mode=indexing
                              tunnel: w238 -> [w244] mode=indexing
                              tunnel: [w242] -> w237 mode=indexing
                              tunnel: w236 -> [w241] mode=indexing
                              tunnel: w235 -> [w240] mode=indexing
                              n176 = Compound Arithmetic op=ADD(w244, w243, w241, w240) -> (w242:dbl)
                            }
                          }
                          frame 1024, Default {
                            n177 = Decimate 1D Array(w254) -> (w252:dbl[], w253:dbl[], w250:dbl[], w249:dbl[], w248:dbl[], w247:dbl[], w246:dbl[], w245:dbl[])
                            n178 = for {
                              tunnel: w253 -> [w262] mode=indexing
                              tunnel: w252 -> [w263] mode=indexing
                              tunnel: [w261] -> w251 mode=indexing
                              tunnel: w250 -> [w260] mode=indexing
                              tunnel: w249 -> [w259] mode=indexing
                              tunnel: w248 -> [w258] mode=indexing
                              tunnel: w247 -> [w257] mode=indexing
                              tunnel: w246 -> [w256] mode=indexing
                              tunnel: w245 -> [w255] mode=indexing
                              n179 = Compound Arithmetic op=ADD(w263, w262, w260, w259, w258, w257, w256, w255) -> (w261:dbl)
                            }
                          }
                        }
                        "变量：显示数据" <- w199
                        n180 = Array Max & Min(array=w199) -> (max value=w204:dbl)  [unwired: 3 out]
                        n181 = Initialize Array(nan ("元素"), w205) -> (w224:dbl[])
                        n182 = Build Array(w199, w224) -> (w225:dbl[][])
                        n183 = Multiply(x=w204, y=1.1) -> (x*y=w202:dbl)
                        n184 = local write "显示：波形图"(w225) -> ()
                        n185 = local write "显示：波形图_预览"(w225) -> ()
                        n186 = local write "变量：图像缓存数组"(w225) -> ()
                        n187 = property on="显示：波形图" class="WFGraph (严格)"("YScale.Maximum"=w202, "YScale.Minimum"=0.0 ("Y标尺.范围:最小值")) -> ()  [unwired: 2 in, 2 out]
                        n188 = property on="显示：波形图_预览" class="WFGraph (严格)"("YScale.Maximum"=w202, "YScale.Minimum"=0.0 ("Y标尺.范围:最小值")) -> ()  [unwired: 2 in, 2 out]
                      }
                      frame #1 {
                        w266 = T5 {"X"=0.0, "Y"=0.0} ("游标.游标位置")
                        n189 = local read "设置：幅度谱总道数"() -> (w265:u32)
                        n190 = property on="显示：波形图_预览" class="WFGraph (严格)"("Cursor.Cursor Position"=w266, "XScale.Maximum"=w265, "XScale.Minimum"=0.0 ("X标尺.范围:最小值")) -> ()  [unwired: 2 in, 2 out]
                        n191 = property on="显示：波形图" class="WFGraph (严格)"("XScale.Maximum"=w265, "XScale.Minimum"=0.0 ("X标尺.范围:最小值"), "Cursor.Cursor Position"=w266, "ActPaletteTool"=0 ("选板:活动工具"), "Cursor.Cursor Plot"=0 ("游标.游标关联曲线"), "Active Plot"=u32 1 ("活动曲线"), "Plot.Visible?"=TRUE ("曲线.可见")) -> ()  [unwired: 2 in, 2 out]
                      }
                    }
                  }
                }
              }
              frame True {
              }
            }
          }
          event "按钮_保存": Value Change {
            n192 = event-data() -> ()  [unwired: 1 in, 6 out]
            n193 = call "MCA_SaveDialog.vi"() -> ("保存数据文件至： 2"=w273:path, "数据文件名称： 2"=w272:string, "是否取消？"=w274:bool)  [unwired: 9 in]
            n194 = case shown="假" w274 {
              tunnel: w273 -> [w304 _]
              tunnel: w272 -> [w305 _]
              frame False {
                n195 = local read "显示：列表显示内容"() -> (w298:string[])
                n196 = Strip Path(path=w304) -> (stripped path=w277:path)  [unwired: 1 out]
                n197 = property on="列表框" class="MCListbox (严格)"() -> ("ItemNames"=w296:string[][])  [unwired: 2 in, 2 out]
                n198 = Concatenate Strings(w305, ".txt" ("字符串")) -> (w278:string)
                n199 = TDMS Open(5:FALSE ("创建索引文件？(T)"), 10:T7."create or replace" ("操作(0:open)"), 11:w304) -> (0:w288:errorcluster, 3:w299:refnum<k34>)  [unwired: 4 in]
                n200 = Index Array(array=w296, index (col)=0 ("禁用的索引 (列)")) -> (element=w294:string[])  [unwired: 1 in]
                n201 = Replace Array Subset(array=w298, new element=w305, index=0 ("索引")) -> (w293:string[])
                n202 = Build Path(base path=w277, name or relative path=w278) -> (appended path=w276:path)
                n203 = local write "显示：列表显示内容"(w293) -> ()
                n204 = Build Array(w294, w293) -> (w285:string[][])
                n205 = local read "变量：图像缓存数组"() -> (w283:dbl[][])
                n206 = local read "变量：上次测量原始数据"() -> (w284:dbl[])
                n207 = TDMS Write(0:w299, 5:"文件属性" ("组名称输入（无标题）"), 7:string[] ["属性名称", "值"] ("通道名输入（无标题）"), 9:w285, 11:w288) -> (4:w292:refnum<k34>, 15:w287:errorcluster)  [unwired: 1 in, 2 out]
                n208 = Index Array(array=w283, index (row)=0 ("索引 (行)")) -> (element=w281:dbl[])  [unwired: 1 in]
                n209 = TDMS Write(0:w292, 5:"数据" ("组名称输入（无标题）"), 7:"计数", 9:w284, 11:w287) -> (4:w289:refnum<k34>, 15:w286:errorcluster)  [unwired: 1 in, 2 out]
                n210 = call-poly <vilib>:"Write To Spreadsheet File.vi"("transpose? (no:F)"=TRUE, "1D data"=w281, "file path (dialog if empty)"=w276) -> ()  [unwired: 5 in, 1 out]
                n211 = TDMS Close(8:w286, 11:w289) -> ()  [unwired: 2 out]
              }
              frame True {
              }
            }
          }
          event "按钮_设置": Value Change {
            n212 = event-data() -> ()  [unwired: 1 in, 1 out]
            n213 = local read "设置：信号极性（正T）"() -> (w324:bool)
            n214 = local read "设置：幅度谱总道数"() -> (w325:u32)
            n215 = local read "设置：寻峰灵敏度"() -> (w316:i32)
            n216 = local read "设置：甄别前阈值"() -> (w315:u16)
            n217 = local read "设置：甄别后阈值"() -> (w314:u16)
            n218 = local read "设置：测量时间"() -> (w321:u16)
            n219 = local read "设置：刷新频率"() -> (w320:u16)
            n220 = local read "设置 ： 修正文件路径"() -> (w319:path)
            n221 = case shown="1024, 默认" w325 {
              tunnel: [enum32{"1024", "2048", "4096", "8192"}."1024" ("道数") enum32{"1024", "2048", "4096", "8192"}."2048" ("道数") enum32{"1024", "2048", "4096", "8192"}."4096" ("道数") enum32{"1024", "2048", "4096", "8192"}."8192" ("道数")] -> w318
              frame 1024, Default {
              }
              frame 2048 {
              }
              frame 4096 {
              }
              frame 8192 {
              }
            }
            n222 = Select(t=enum32{"正", "负"}."正" ("y"), s=w324, f=enum32{"正", "负"}."负" ("y")) -> (s? t:f=w317:enum32{"正", "负"})
            n223 = call "MCA_ConfigDialog.vi"("测量最多花费的时间（秒）："=w321, "测量数据刷新频率（个/次）："=w320, "数据文件路径"=w319, "道数"=w318, "输入信号的极性："=w317, "寻峰灵敏度："=w316, "甄别前阈值"=w315, "甄别后阈值"=w314) -> ("输入信号极性"=w313:bool, "甄别后阈值 2"=w311:dbl, "甄别前阈值 2"=w312:dbl, "是否取消？"=w326:bool, "道数最大值"=w310:i32, "数据文件路径 2"=w309:path, "寻峰灵敏度： 2"=w308:u32, "测量数据刷新时间（个/次）： 2"=w307:u32, "测量最多花费的时间（秒）： 2"=w306:u32)  [unwired: 11 in]
            n224 = case shown="假" w326 {
              tunnel: w312 -> [w383 _]
              tunnel: w309 -> [w381 _]
              tunnel: w310 -> [w358 _]
              tunnel: w325 -> [w359 _]
              tunnel: w313 -> [w337 _]
              tunnel: w311 -> [w335 _]
              tunnel: w308 -> [w334 _]
              tunnel: w307 -> [w333 _]
              tunnel: w306 -> [w332 _]
              frame False {
                n225 = Divide(x=w359, y=w358) -> (x/y=w351:dbl)
                n226 = local read "变量：感兴区起点道址"() -> (w357:dbl)
                n227 = local read "变量：感兴区终点道址"() -> (w356:dbl)
                n228 = property on="显示：波形图" class="WFGraph (严格)"("XScale.Maximum"=w358, "XScale.Minimum"=0.0 ("X标尺.范围:最小值")) -> ()  [unwired: 2 in, 2 out]
                n229 = Equal?(x=w381, y=path "") -> (x = y?=w380:bool)
                n230 = property on="显示：波形图_预览" class="WFGraph (严格)"("XScale.Maximum"=w358, "XScale.Minimum"=0.0 ("X标尺.范围:最小值")) -> ()  [unwired: 2 in, 2 out]
                n231 = local write "设置：幅度谱总道数"(w358) -> ()
                n232 = local write "设置：信号极性（正T）"(w337) -> ()
                n233 = local write "设置：甄别后阈值"(w335) -> ()
                n234 = local write "设置：甄别前阈值"(w383) -> ()
                n235 = case shown="真" w380 {
                  tunnel: w381 -> [w444 _]
                  tunnel: [w442 w445] -> w347
                  frame False {
                    n236 = call-poly <vilib>:"Read From Spreadsheet File.vi"("transpose (no:F)"=TRUE, "file path (dialog if empty)"=w444) -> ("first row"=w442:dbl[])  [unwired: 5 in, 4 out]
                  }
                  frame True {
                    n237 = local read "MCA道宽修正数组"() -> (w445:ext[])
                  }
                }
                n238 = local write "设置：寻峰灵敏度"(w334) -> ()
                n239 = local write "设置：刷新频率"(w333) -> ()
                n240 = local write "设置：测量时间"(w332) -> ()
                n241 = local write "变量：每次测量计划用时"(w332) -> ()
                n242 = Divide(x=w357, y=w351) -> (x/y=w355:dbl)
                n243 = Divide(x=w356, y=w351) -> (x/y=w354:dbl)
                n244 = property on="显示：波形图" class="WFGraph (严格)"("Active Cursor"=u32 0 ("活动游标")) -> ("Cursor.Cursor X"=w352:dbl)  [unwired: 2 in, 2 out]
                n245 = local write "变量：感兴区起点道址"(w355) -> ()
                n246 = local write "变量：感兴区终点道址"(w354) -> ()
                n247 = local write "MCA道宽修正数组"(w347) -> ()
                n248 = Divide(x=w352, y=w351) -> (x/y=w350:dbl)
                n249 = local read "变量：原始数据"() -> (w336:dbl[])
                n250 = Divide(x=8192.0, y=w358) -> (x/y=w360:dbl)
                n251 = property on="显示：波形图" class="WFGraph (严格)"("Cursor.Cursor X"=w350) -> ()  [unwired: 2 in, 2 out]
                n252 = property on="显示：波形图_预览" class="WFGraph (严格)"("Cursor.Cursor X"=w350) -> ()  [unwired: 2 in, 2 out]
                n253 = local read "设置：寻峰灵敏度"() -> (w364:i32)
                n254 = local read "设置：信号极性（正T）"() -> (w346:bool)
                n255 = local read "设置：幅度谱总道数"() -> (w343:u32)
                n256 = local read "设置：测量时间"() -> (w368:u16)
                n257 = local read "设置：刷新频率"() -> (w367:u16)
                n258 = local read "设置：甄别前阈值"() -> (w366:u16)
                n259 = local read "设置：甄别后阈值"() -> (w365:u16)
                n260 = stacked-sequence {
                  tunnel: w336 -> [w389 _]
                  tunnel: w360 -> [w388 _]
                  frame #0 {
                    n261 = case shown="8" w388 {
                      tunnel: w389 -> [w392 w396 w405 w420]
                      tunnel: [w392 w393 w402 w417] -> w386
                      frame 1, Default {
                      }
                      frame 2 {
                        n262 = Decimate 1D Array(w396) -> (w394:dbl[], w395:dbl[])
                        n263 = for {
                          tunnel: w395 -> [w398] mode=indexing
                          tunnel: w394 -> [w399] mode=indexing
                          tunnel: [w397] -> w393 mode=indexing
                          n264 = Add(x=w399, y=w398) -> (x+y=w397:dbl)
                        }
                      }
                      frame 4 {
                        n265 = Decimate 1D Array(w405) -> (w403:dbl[], w404:dbl[], w401:dbl[], w400:dbl[])
                        n266 = for {
                          tunnel: w404 -> [w409] mode=indexing
                          tunnel: w403 -> [w410] mode=indexing
                          tunnel: [w408] -> w402 mode=indexing
                          tunnel: w401 -> [w407] mode=indexing
                          tunnel: w400 -> [w406] mode=indexing
                          n267 = Compound Arithmetic op=ADD(w410, w409, w407, w406) -> (w408:dbl)
                        }
                      }
                      frame 8 {
                        n268 = Decimate 1D Array(w420) -> (w418:dbl[], w419:dbl[], w416:dbl[], w415:dbl[], w414:dbl[], w413:dbl[], w412:dbl[], w411:dbl[])
                        n269 = for {
                          tunnel: w419 -> [w428] mode=indexing
                          tunnel: w418 -> [w429] mode=indexing
                          tunnel: [w427] -> w417 mode=indexing
                          tunnel: w416 -> [w426] mode=indexing
                          tunnel: w415 -> [w425] mode=indexing
                          tunnel: w414 -> [w424] mode=indexing
                          tunnel: w413 -> [w423] mode=indexing
                          tunnel: w412 -> [w422] mode=indexing
                          tunnel: w411 -> [w421] mode=indexing
                          n270 = Compound Arithmetic op=ADD(w429, w428, w426, w425, w424, w423, w422, w421) -> (w427:dbl)
                        }
                      }
                    }
                    n271 = for {
                      tunnel: w386 -> [_] mode=indexing
                      tunnel: [nan] -> w390 mode=indexing
                    }
                    n272 = local write "变量：显示数据"(w386) -> ()
                    n273 = Build Array(w386, w390) -> (w387:dbl[][])
                    n274 = local write "显示：波形图"(w387) -> ()
                    n275 = local write "显示：波形图_预览"(w387) -> ()
                    n276 = local write "变量：图像缓存数组"(w387) -> ()
                  }
                  frame #1 {
                    n277 = local read "变量：图像缓存数组"() -> (w439:dbl[][])
                    n278 = Index Array(array=w439, index (row)=0 ("索引 (行)")) -> (element=w440:dbl[])  [unwired: 1 in]
                    n279 = Array Max & Min(array=w440) -> (max value=w433:dbl)  [unwired: 3 out]
                    n280 = Multiply(x=w433, y=1.1) -> (x*y=w436:dbl)
                    n281 = Less?(x=w436, y=10.0) -> (x < y?=w438:bool)
                    n282 = Select(t=10.0, s=w438, f=w436) -> (s? t:f=w430:dbl)
                    n283 = property on="显示：波形图_预览" class="WFGraph (严格)"("YScale.Maximum"=w430, "YScale.Minimum"=0.0 ("Y标尺.范围:最小值")) -> ()  [unwired: 2 in, 2 out]
                    n284 = property on="显示：波形图" class="WFGraph (严格)"("YScale.Maximum"=w430, "YScale.Minimum"=0.0 ("X标尺.范围:最小值")) -> ()  [unwired: 2 in, 2 out]
                  }
                }
                n285 = case shown="假" w346 {
                  tunnel: ["负" ("字符串") "正" ("字符串")] -> w344
                  frame False {
                  }
                  frame True {
                  }
                }
                n286 = Number To Decimal String(number=w364) -> (decimal integer string=w339:string)  [unwired: 1 in]
                n287 = Number To Decimal String(number=w368) -> (decimal integer string=w372:string)  [unwired: 1 in]
                n288 = Number To Decimal String(number=w367) -> (decimal integer string=w377:string)  [unwired: 1 in]
                n289 = Number To Decimal String(number=w366) -> (decimal integer string=w349:string)  [unwired: 1 in]
                n290 = Number To Decimal String(number=w365) -> (decimal integer string=w348:string)  [unwired: 1 in]
                n291 = Number To Decimal String(number=w343) -> (decimal integer string=w341:string)  [unwired: 1 in]
                n292 = Concatenate Strings(w372, "秒" ("字符串")) -> (w373:string)
                n293 = Concatenate Strings(w377, "个/次" ("字符串")) -> (w379:string)
                n294 = local read "显示：列表显示内容"() -> (w370:string[])
                n295 = Replace Array Subset(array=w370, new element #1=w373, index #1=1 ("索引"), new element #2=w379, index #2=2 ("索引"), new element #3=w349, index #3=3 ("索引"), new element #4=w348, index #4=4 ("索引"), new element #5=w344, index #5=5 ("索引"), new element #6=w341, index #6=6 ("索引"), new element #7=w339, index #7=18 ("索引")) -> (w338:string[])
                n296 = local write "显示：列表显示内容"(w338) -> ()
              }
              frame True {
              }
            }
          }
          event "按钮_对数": Value Change {
            n297 = event-data() -> ()  [unwired: 1 in, 6 out]
            n298 = local read "按钮_对数"() -> (w446:bool)
            n299 = case shown="真" w446 {
              frame False {
                w448 = u8 0 ("Y标尺.映射模式")
                n300 = property on="显示：波形图" class="WFGraph (严格)"("YScale.Mapping Mode"=w448) -> ()  [unwired: 2 in, 2 out]
                n301 = property on="显示：波形图_预览" class="WFGraph (严格)"("YScale.Mapping Mode"=w448) -> ()  [unwired: 2 in, 2 out]
              }
              frame True {
                w449 = u8 1 ("Y标尺.映射模式")
                n302 = property on="显示：波形图" class="WFGraph (严格)"("YScale.Mapping Mode"=w449) -> ()  [unwired: 2 in, 2 out]
                n303 = property on="显示：波形图_预览" class="WFGraph (严格)"("YScale.Mapping Mode"=w449) -> ()  [unwired: 2 in, 2 out]
              }
            }
          }
          event "按钮_游标": Value Change {
            # "游标显示时，左右移按钮才可以用才可用"
            n304 = event-data() -> ()  [unwired: 1 in, 1 out]
            n305 = property on="显示：波形图" class="WFGraph (严格)"("Active Cursor"=u32 0 ("活动游标")) -> (error out=w451:errorcluster)  [unwired: 2 in, 1 out]
            n306 = property on="显示：波形图" class="WFGraph (严格)"(error in=w451) -> (error out=w453:errorcluster, "Cursor.Visible"=w461:bool)  [unwired: 1 in, 1 out]
            n307 = property on="显示：波形图_预览" class="WFGraph (严格)"(error in=w451) -> (error out=w452:errorcluster, "Cursor.Visible"=w456:bool)  [unwired: 1 in, 1 out]
            n308 = Not(x=w461) -> (.not. x?=w450:bool)
            n309 = Not(x=w456) -> (.not. x?=w455:bool)
            n310 = property on="显示：波形图" class="WFGraph (严格)"(error in=w453, "Cursor.Visible"=w450) -> ()  [unwired: 1 in, 2 out]
            n311 = property on="显示：波形图_预览" class="WFGraph (严格)"(error in=w452, "Cursor.Visible"=w455) -> ()  [unwired: 1 in, 2 out]
            n312 = Select(t="显示", s=w450, f="隐藏") -> (s? t:f=→"状态栏_游标状态":string)
            n313 = case shown="真" w450 {
              frame False {
                w462 = T6."Disabled and Grayed Out" ("禁用")
                w463 = ""
                n314 = local write "状态栏_游标道址"(w463) -> ()
                n315 = local write "状态栏_游标计数"(w463) -> ()
                n316 = property on="按钮_右移" class="Bool"("DisabledEnum"=w462) -> ()  [unwired: 2 in, 2 out]
                n317 = property on="按钮_左移" class="Bool"("DisabledEnum"=w462) -> ()  [unwired: 2 in, 2 out]
              }
              frame True {
                w466 = T6."Enabled" ("禁用")
                n318 = property on="显示：波形图" class="WFGraph (严格)"() -> (error out=w465:errorcluster, "Cursor.Cursor X"=w472:dbl)  [unwired: 2 in, 1 out]
                n319 = Number To Decimal String(number=w472) -> (decimal integer string=w473:string)  [unwired: 1 in]
                n320 = local write "状态栏_游标道址"(w473) -> ()
                n321 = property on="显示：波形图" class="WFGraph (严格)"(error in=w465, "Cursor.Cursor Plot"=0 ("游标.游标关联曲线")) -> ("Cursor.Cursor Y"=w468:dbl)  [unwired: 1 in, 2 out]
                n322 = property on="按钮_右移" class="Bool"("DisabledEnum"=w466) -> ()  [unwired: 2 in, 2 out]
                n323 = property on="按钮_左移" class="Bool"("DisabledEnum"=w466) -> ()  [unwired: 2 in, 2 out]
                n324 = Number To Decimal String(number=w468) -> (decimal integer string=w470:string)  [unwired: 1 in]
                n325 = Equal?(x=w470, y="NaN") -> (x = y?=w467:bool)
                n326 = case shown="假" w467 {
                  tunnel: w470 -> [w474 _]
                  tunnel: [w474 "0"] -> w471
                  frame False {
                  }
                  frame True {
                  }
                }
                n327 = local write "状态栏_游标计数"(w471) -> ()
              }
            }
          }
          event "按钮_放大": Value Change {
            w480 = 0
            n328 = event-data() -> ()  [unwired: 1 in, 6 out]
            n329 = local read "变量：感兴区起点道址"() -> (w492:dbl)
            n330 = local read "变量：感兴区终点道址"() -> (w489:dbl)
            n331 = Subtract(x=w492, y=w489) -> (x-y=w481:dbl)
            n332 = Divide(x=w481, y=2.0) -> (x/y=w490:dbl)
            n333 = Add(x=w490, y=w489) -> (x+y=w488:dbl)
            n334 = local read "设置：幅度谱总道数"() -> (w479:u32)
            n335 = Add(x=w481, y=w488) -> (x+y=w487:dbl)
            n336 = Subtract(x=w488, y=w481) -> (x-y=w482:dbl)
            n337 = property on="按钮_放大" class="Bool"("DisabledEnum"=T6."Disabled and Grayed Out" ("禁用")) -> ()  [unwired: 2 in, 2 out]
            n338 = Greater?(x=w480, y=w487) -> (0:w486:bool)
            n339 = Less?(x=w482, y=w479) -> (x < y?=w484:bool)
            n340 = Select(t=w480, s=w486, f=w487) -> (s? t:f=w485:dbl)
            n341 = Select(t=w482, s=w484, f=w479) -> (s? t:f=w483:dbl)
            n342 = To Quad Integer(1:w485) -> (0:w477:i64)
            n343 = To Quad Integer(1:w483) -> (0:w478:i64)
            n344 = property on="显示：波形图" class="WFGraph (严格)"("XScale.Maximum"=w478, "XScale.Minimum"=w477) -> ()  [unwired: 2 in, 2 out]
          }
          event "按钮_还原": Value Change {
            w505 = 0.0 ("变量：起点道址")
            w494 = ""
            # "列表复位"
            # "图像数据复位"
            # "游标起点、终点和标记复位"
            n345 = event-data() -> ()  [unwired: 1 in, 1 out]
            n346 = property on="显示：波形图" class="WFGraph (严格)"("Active Cursor"=u32 1 ("活动游标"), "Cursor.Visible"=FALSE ("游标.可见"), "Cursor.Cursor Plot"=1 ("游标.游标关联曲线"), "Cursor.Cursor Name"="" ("游标.游标名")) -> (error out=w496:errorcluster)  [unwired: 2 in, 1 out]
            n347 = local read "设置：幅度谱总道数"() -> (w510:u32)
            n348 = local read "显示：列表显示内容"() -> (w509:string[])
            n349 = property on="显示：波形图_预览" class="WFGraph (严格)"("Cursor.Cursor Position"=T5 {"X"=0.0, "Y"=0.0} ("游标.游标位置")) -> ()  [unwired: 2 in, 2 out]
            n350 = property on="显示：波形图" class="WFGraph (严格)"(error in=w496, "XScale.Maximum"=w510, "XScale.Minimum"=0.0 ("X标尺.范围:最小值"), "Cursor.Cursor Position"=T5 {"X"=0.0, "Y"=0.0} ("游标.游标位置"), "ActPaletteTool"=0 ("选板:活动工具"), "Cursor.Cursor Plot"=0 ("游标.游标关联曲线")) -> ()  [unwired: 1 in, 2 out]
            n351 = Replace Array Subset(array=w509, new element #1=w494, index #1=12 ("索引"), new element #2=w494, index #2=13 ("索引"), new element #3=w494, index #3=14 ("索引"), new element #4=w494, index #4=15 ("索引"), new element #5=w494, index #5=16 ("索引"), new element #6=w494, index #6=17 ("索引")) -> (w508:string[])
            n352 = local write "显示：列表显示内容"(w508) -> ()
            n353 = local read "变量：图像缓存数组"() -> (w495:dbl[][])
            n354 = local write "变量：感兴区起点道址"(w505) -> ()
            n355 = local write "变量：感兴区终点道址"(w505) -> ()
            n356 = local write "显示：波形图_预览"(w495) -> ()
            n357 = local write "显示：波形图"(w495) -> ()
          }
          event "按钮_左移": Value Change {
            n358 = event-data() -> ()  [unwired: 1 in, 6 out]
            n359 = property on="显示：波形图" class="WFGraph (严格)"("Active Cursor"=u32 0 ("活动游标")) -> ("Cursor.Cursor X"=w517:dbl)  [unwired: 2 in, 2 out]
            n360 = property on="显示：波形图" class="WFGraph (严格)"() -> ("XScale.Minimum"=w519:dbl)  [unwired: 2 in, 2 out]
            n361 = Decrement(x=w517) -> (x-1=w520:dbl)
            n362 = Greater?(x=w520, y=w519) -> (0:w521:bool)
            n363 = case shown="真" w521 {
              tunnel: w520 -> [_ w523]
              frame False {
              }
              frame True {
                n364 = property on="显示：波形图" class="WFGraph (严格)"("Cursor.Cursor X"=w523) -> ()  [unwired: 2 in, 2 out]
              }
            }
          }
          event "显示：波形图": Mouse Down {
            # "解决“标记后出现上一次寻峰的结果”的问题"
            n365 = event-data() -> ()  [unwired: 1 in, 8 out]
            n366 = property on="显示：波形图" class="WFGraph (严格)"("Active Cursor"=u32 0 ("活动游标")) -> (error out=w526:errorcluster, "Cursor.Cursor X"=w525:dbl)  [unwired: 2 in, 1 out]
            n367 = property on="显示：波形图" class="WFGraph (严格)"(error in=w526, "Active Cursor"=u32 1 ("活动游标"), "Cursor.Cursor X"=0.0 ("游标.游标位置:游标X坐标"), "Cursor.Cursor Name"="" ("游标.游标名")) -> ()  [unwired: 1 in, 2 out]
            n368 = local write "变量：感兴区起点道址"(w525) -> ()
          }
          event "显示：波形图": Mouse Up {
            n369 = event-data() -> ()  [unwired: 1 in, 8 out]
            n370 = flat-sequence {
              frame #0 {
                n371 = property on="显示：波形图" class="WFGraph (严格)"("Active Cursor"=u32 0 ("活动游标")) -> ("Cursor.Cursor X"=w532:dbl)  [unwired: 2 in, 2 out]
                n372 = local write "变量：感兴区终点道址"(w532) -> ()
              }
              frame #1 {
                n373 = local read "变量：感兴区起点道址"() -> (w536:dbl)
                n374 = local read "变量：感兴区终点道址"() -> (w535:dbl)
                n375 = Equal?(x=w536, y=w535) -> (x = y?=w534:bool)
                n376 = case shown="假" w534 {
                  tunnel: w535 -> [w541 _]
                  tunnel: w536 -> [w542 _]
                  frame False {
                    # "若起点比终点大，起点和中间交换"
                    n377 = local read "状态：停止变量"() -> (w538:bool)
                    n378 = Greater?(x=w542, y=w541) -> (0:w543:bool)
                    n379 = case shown="假" w543 {
                      tunnel: w542 -> [w546 w548]
                      tunnel: w541 -> [w545 w547]
                      tunnel: [w546 w547] -> w540
                      tunnel: [w545 w548] -> w539
                      frame False {
                        # "起点比终点小，不变"
                      }
                      frame True {
                      }
                    }
                    n380 = case shown="真" w538 {
                      frame False {
                      }
                      frame True {
                        n381 = property on="按钮_寻峰" class="Bool"("DisabledEnum"=T6."Enabled" ("禁用")) -> ()  [unwired: 2 in, 2 out]
                      }
                    }
                    n382 = local write "变量：感兴区起点道址"(w540) -> ()
                    n383 = local write "变量：感兴区终点道址"(w539) -> ()
                    n384 = property on="按钮_放大" class="Bool"("DisabledEnum"=T6."Enabled" ("禁用")) -> ()  [unwired: 2 in, 2 out]
                  }
                  frame True {
                  }
                }
              }
            }
          }
          event "按钮_右移": Value Change {
            n385 = event-data() -> ()  [unwired: 1 in, 6 out]
            n386 = property on="显示：波形图" class="WFGraph (严格)"("Active Cursor"=u32 0 ("活动游标")) -> ("Cursor.Cursor X"=w549:dbl)  [unwired: 2 in, 2 out]
            n387 = property on="显示：波形图" class="WFGraph (严格)"() -> ("XScale.Maximum"=w551:dbl)  [unwired: 2 in, 2 out]
            n388 = Increment(x=w549) -> (x+1=w552:dbl)
            n389 = Less Or Equal?(x=w552, y=w551) -> (x <= y?=w553:bool)
            n390 = case shown="真" w553 {
              tunnel: w552 -> [_ w555]
              frame False {
              }
              frame True {
                n391 = property on="显示：波形图" class="WFGraph (严格)"("Cursor.Cursor X"=w555) -> ()  [unwired: 2 in, 2 out]
              }
            }
          }
          event Value Change {
            n392 = event-data() -> ()  [unwired: 1 in, 1 out]
            n393 = stacked-sequence {
              frame #0 {
                n394 = local read "变量：感兴区起点道址"() -> (w572:dbl)
                n395 = local read "变量：感兴区终点道址"() -> (w571:dbl)
                n396 = local read "变量：图像缓存数组"() -> (w570:dbl[][])
                n397 = call "MCA_Confirming Interested area Dialog.vi"("终点道址："=w571, "起点道址："=w572) -> ("终点道址： 2"=w560:u32, "起点道址： 2"=w562:u32)
                n398 = Index Array(array=w570, index (row)=0 ("索引 (行)")) -> (element=w567:dbl[])  [unwired: 1 in]
                n399 = call "一线双色计算.vi"("输入一维数组"=w567, "right corsor"=w560, "left corsor"=w562) -> ("输出波形数组"=w569:dbl[][])
                n400 = local write "变量：感兴区终点道址"(w560) -> ()
                n401 = local write "显示：波形图_预览"(w569) -> ()
                n402 = local write "显示：波形图"(w569) -> ()
                n403 = local write "变量：感兴区起点道址"(w562) -> ()
                n404 = local read "显示：列表显示内容"() -> (w565:string[])
                n405 = Number To Fractional String(number=w560, precision (6)=i16 0 ("精度(6)")) -> (F-format string=w559:string)  [unwired: 2 in]
                n406 = Number To Fractional String(number=w562, precision (6)=i16 0 ("精度(6)")) -> (F-format string=w561:string)  [unwired: 2 in]
                n407 = Replace Array Subset(array=w565, new element #1=w561, index #1=12 ("索引"), new element #2=w559, index #2=13 ("索引")) -> (w566:string[])
                n408 = local write "显示：列表显示内容"(w566) -> ()
              }
              frame #1 {
                n409 = local read "变量：图像缓存数组"() -> (w623:dbl[][])
                n410 = property on="按钮_寻峰" class="Bool"("DisabledEnum"=T6."Disabled and Grayed Out" ("禁用")) -> ()  [unwired: 2 in, 2 out]
                n411 = local read "变量：感兴区起点道址"() -> (w621:dbl)
                n412 = local read "变量：感兴区终点道址"() -> (w620:dbl)
                n413 = Index Array(array=w623, index (row)=0 ("索引 (行)")) -> (element=w619:dbl[])  [unwired: 1 in]
                n414 = for {
                  tunnel: w619 -> [w628] mode=indexing
                  tunnel: w621 -> [w633]
                  tunnel: w620 -> [w626]
                  tunnel: [w627] -> w582 mode=indexing
                  tunnel: [w625] -> w583 mode=indexing
                  i -> [w625]
                  n415 = Greater Or Equal?(x=w625, y=w633) -> (x >= y?=w632:bool)
                  n416 = Less Or Equal?(x=w625, y=w626) -> (x <= y?=w631:bool)
                  n417 = And(x=w632, y=w631) -> (x .and. y?=w630:bool)
                  n418 = Select(t=w628, s=w630, f=0.0) -> (s? t:f=w627:dbl)
                }
                n419 = Array Max & Min(array=w582) -> (max value=w590:dbl)  [unwired: 3 out]
                n420 = Multiply(x=w590, y=0.85) -> (x*y=w591:dbl)
                n421 = call <vilib>:"Gaussian Peak Fit.vi"("Y"=w582, "X"=w583) -> ("center"=→"center":dbl, "standard deviation"=w580:dbl)  [unwired: 7 in, 5 out]
                n422 = call <vilib>:"Peak Detector.vi"("peaks/valleys"=enum32{"Peaks", "Valleys"}."Peaks", "width"="设置：寻峰灵敏度", "threshold"=w591, "X"=w582) -> ("Amplitudes"=w585:dbl[], "Locations"=w588:dbl[])  [unwired: 3 in, 3 out]
                n423 = Multiply(x=2.355, y=w580) -> (x*y=w575:dbl)
                "结果：半高宽" <- w575
                n424 = Index Array(array=w588, index=0 ("索引")) -> (element=w576:dbl)
                "结果：峰位" <- w576
                n425 = Index Array(array=w585, index=0 ("索引")) -> ()  [unwired: 1 out]
                n426 = Add Array Elements(numeric array=w582) -> (sum=w573:dbl)
                "结果：净面积" <- w573
                n427 = Divide(x=w575, y=w576) -> (x/y=w600:dbl)
                n428 = Equal?(x=w576, y=0.0) -> (x = y?=w578:bool)
                n429 = Multiply(x=w600, y=100.0) -> (x*y=w598:dbl)
                n430 = Number To Fractional String(number=w576, precision (6)=i16 2 ("精度(6)")) -> (F-format string=w577:string)  [unwired: 2 in]
                n431 = Number To Fractional String(number=w575, precision (6)=i16 2 ("精度(6)")) -> (F-format string=w605:string)  [unwired: 2 in]
                n432 = Number To Fractional String(number=w573, precision (6)=i16 0 ("精度(6)")) -> (F-format string=w602:string)  [unwired: 2 in]
                n433 = local read "显示：列表显示内容"() -> (w609:string[])
                n434 = case shown="真" w578 {
                  frame False {
                  }
                  frame True {
                    n435 = One Button Dialog(message="    未寻到有效峰值！请设置合适的寻峰灵敏度后，重新寻峰！    \n（寻峰灵敏度请按工具栏“设置”按钮，“寻峰设置”标签设置）" ("消息")) -> ()  [unwired: 1 in, 1 out]
                  }
                }
                n436 = Number To Fractional String(number=w598, precision (6)=i16 2 ("精度(6)")) -> (F-format string=w596:string)  [unwired: 2 in]
                n437 = Number To Fractional String(number=w576, precision (6)=i16 2 ("精度(6)")) -> (F-format string=w613:string)  [unwired: 2 in]
                n438 = Concatenate Strings(w596, "%" ("字符串")) -> (w594:string)
                n439 = property on="显示：波形图" class="WFGraph (严格)"("Active Cursor"=u32 1 ("活动游标"), "Cursor.Cursor X"=w576, "Cursor.Visible"=TRUE ("游标.可见"), "Cursor.Cursor Plot"=1 ("游标.游标关联曲线"), "Cursor.Cursor Name"=w613) -> (error out=w615:errorcluster)  [unwired: 2 in, 1 out]
                n440 = Replace Array Subset(array=w609, new element #1=w577, index #1=14 ("索引"), new element #2=w605, index #2=15 ("索引"), new element #3=w602, index #3=16 ("索引"), new element #4=w594, index #4=17 ("索引")) -> (w608:string[])
                n441 = local write "显示：列表显示内容"(w608) -> ()
                n442 = property on="显示：波形图" class="WFGraph (严格)"(error in=w615, "Active Cursor"=u32 0 ("活动游标")) -> ()  [unwired: 1 in, 2 out]
              }
            }
          }
          event Key Down {
            n443 = event-data() -> ("VKey"=w634:T8)  [unwired: 1 in, 5 out]
            n444 = case shown="\"Right\"" w634 {
              frame "Left" {
                n445 = property on="显示：波形图" class="WFGraph (严格)"() -> ("Cursor.Visible"=w636:bool)  [unwired: 2 in, 2 out]
                n446 = case shown="真" w636 {
                  frame False {
                  }
                  frame True {
                    n447 = property on="显示：波形图" class="WFGraph (严格)"("Active Cursor"=u32 0 ("活动游标")) -> (error out=w637:errorcluster, "Cursor.Cursor X"=w638:dbl)  [unwired: 2 in, 1 out]
                    n448 = property on="显示：波形图" class="WFGraph (严格)"() -> ("XScale.Minimum"=w640:dbl)  [unwired: 2 in, 2 out]
                    n449 = Decrement(x=w638) -> (x-1=w641:dbl)
                    n450 = Greater?(x=w641, y=w640) -> (0:w642:bool)
                    n451 = case shown="真" w642 {
                      tunnel: w641 -> [_ w643]
                      tunnel: w637 -> [_ _]
                      frame False {
                      }
                      frame True {
                        n452 = property on="显示：波形图" class="WFGraph (严格)"("Cursor.Cursor X"=w643) -> ()  [unwired: 2 in, 2 out]
                      }
                    }
                  }
                }
              }
              frame "Right" {
                n453 = property on="显示：波形图" class="WFGraph (严格)"() -> ("Cursor.Visible"=w644:bool)  [unwired: 2 in, 2 out]
                n454 = case shown="真" w644 {
                  frame False {
                  }
                  frame True {
                    n455 = property on="显示：波形图" class="WFGraph (严格)"("Active Cursor"=u32 0 ("活动游标")) -> (error out=w645:errorcluster, "Cursor.Cursor X"=w646:dbl)  [unwired: 2 in, 1 out]
                    n456 = property on="显示：波形图" class="WFGraph (严格)"() -> ("XScale.Maximum"=w648:dbl)  [unwired: 2 in, 2 out]
                    n457 = Increment(x=w646) -> (x+1=w649:dbl)
                    n458 = Less Or Equal?(x=w649, y=w648) -> (x <= y?=w650:bool)
                    n459 = case shown="真" w650 {
                      tunnel: w649 -> [_ w651]
                      tunnel: w645 -> [_ _]
                      frame False {
                      }
                      frame True {
                        n460 = property on="显示：波形图" class="WFGraph (严格)"("Cursor.Cursor X"=w651) -> ()  [unwired: 2 in, 2 out]
                      }
                    }
                  }
                }
              }
              frame "ASCII", Default {
              }
            }
          }
        }
      }
      frame "完成" {
      }
    }
  }
  n461 = while {
    stop <- w654 stop-if-true
    n462 = event shown="[3] \"按钮_开始\": 值改变" {
      selector: _ -> [_ _ _ _]
      dyn-events: _ -> [_ _ _ _]
      timeout: _ -> [_ _ _ _]
      tunnel: [_ _ TRUE _] -> w654
      event Timeout {
        n463 = event-data() -> ()  [unwired: 1 in, 1 out]
      }
      event "按钮_复位": Value Change {
        w676 = 0.0 ("变量：起点道址")
        w660 = 0.0 ("已测量时间")
        w681 = ""
        w668 = T6."Disabled and Grayed Out" ("禁用")
        n464 = event-data() -> ()  [unwired: 1 in, 1 out]
        n465 = local read "变量：每次测量计划用时"() -> (w656:u16)
        n466 = local read "显示：列表显示内容"() -> (w667:string[])
        n467 = property on="显示：波形图" class="WFGraph (严格)"("Active Cursor"=u32 1 ("活动游标"), "Cursor.Visible"=FALSE ("游标.可见"), "Cursor.Cursor Plot"=1 ("游标.游标关联曲线"), "Cursor.Cursor Name"="" ("游标.游标名")) -> ()  [unwired: 2 in, 2 out]
        n468 = Number To Decimal String(number=w656) -> (decimal integer string=w657:string)  [unwired: 1 in]
        n469 = property on="按钮_开始" class="Bool"("DisabledEnum"=T6."Enabled" ("禁用")) -> ()  [unwired: 2 in, 2 out]
        n470 = Concatenate Strings(w657, "秒" ("字符串")) -> (w655:string)
        n471 = Replace Array Subset(array=w667, new element #1="未命名" ("新元素/子数组"), index #1=0 ("索引"), new element #2=w681, index #2=7 ("索引"), new element #3=w681, index #3=8 ("索引"), new element #4=w681, index #4=9 ("索引"), new element #5=w681, index #5=10 ("索引"), new element #6=w681, index #6=11 ("索引"), new element #7=w681, index #7=12 ("索引"), new element #8=w681, index #8=13 ("索引"), new element #9=w681, index #9=14 ("索引"), new element #10=w681, index #10=15 ("索引"), new element #11=w681, index #11=16 ("索引"), new element #12=w681, index #12=17 ("索引"), new element #13=w655, index #13=1 ("索引")) -> (w694:string[])
        n472 = local write "显示：列表显示内容"(w694) -> ()
        n473 = local write "变量 ： 上次测量总计数"(w660) -> ()
        n474 = local write "变量 : 实时总计数"(w660) -> ()
        n475 = local write "状态：已测时间"(w660) -> ()
        n476 = local write "状态：本次测量和上次未完成测量时间和"(w660) -> ()
        n477 = local write "状态：上次未完成测试的已测时间"(w660) -> ()
        n478 = local write "状态：本次测试已测时间"(w660) -> ()
        n479 = local read "变量：每次测量计划用时"() -> (w661:u16)
        n480 = property on="按钮_寻峰" class="Bool"("DisabledEnum"=w668) -> ()  [unwired: 2 in, 2 out]
        n481 = property on="按钮_右移" class="Bool"("DisabledEnum"=w668) -> ()  [unwired: 2 in, 2 out]
        n482 = property on="按钮_左移" class="Bool"("DisabledEnum"=w668) -> ()  [unwired: 2 in, 2 out]
        n483 = property on="按钮_放大" class="Bool"("DisabledEnum"=w668) -> ()  [unwired: 2 in, 2 out]
        n484 = property on="按钮_停止" class="Bool (严格)"("DisabledEnum"=w668) -> ()  [unwired: 2 in, 2 out]
        n485 = local read "设置：幅度谱总道数"() -> (w696:u32)
        n486 = local write "状态栏_计数率"(T3 "" ("状态栏_计数率")) -> ()
        n487 = local write "状态栏_测量状态"(T3 "停止" ("状态栏_测量状态")) -> ()
        n488 = local write "设置：测量时间"(w661) -> ()
        n489 = local write "变量：感兴区起点道址"(w676) -> ()
        n490 = local write "变量：感兴区终点道址"(w676) -> ()
        n491 = property on="显示：波形图" class="WFGraph (严格)"("XScale.Maximum"=w696, "XScale.Minimum"=0.0 ("X标尺.范围:最小值"), "Cursor.Cursor Position"=T5 {"X"=0.0, "Y"=0.0} ("游标.游标位置"), "Active Cursor"=0 ("游标.游标关联曲线")) -> (error out=w698:errorcluster, "Cursor.Visible"=w673:bool)  [unwired: 2 in, 1 out]
        n492 = case shown="真" w673 {
          frame False {
          }
          frame True {
            w707 = "0"
            n493 = local write "状态栏_游标道址"(w707) -> ()
            n494 = local write "状态栏_游标计数"(w707) -> ()
          }
        }
        n495 = Initialize Array(nan ("元素"), 8192 ("维数大小")) -> (w669:dbl[])
        n496 = Initialize Array(0.0 ("元素"), 8192 ("维数大小")) -> (w672:dbl[])
        n497 = Initialize Array(nan ("元素"), 8192 ("维数大小")) -> (w662:dbl[])
        n498 = local write "变量：上次测量原始数据"(w672) -> ()
        n499 = Build Array(w669, w669) -> (w706:dbl[][])
        n500 = property on="显示：波形图_预览" class="WFGraph (严格)"(error in=w698, "XScale.Maximum"=w696, "XScale.Minimum"=0.0 ("X标尺.范围:最小值"), "Cursor.Cursor Position"=T5 {"X"=0.0, "Y"=0.0} ("游标.游标位置")) -> ()  [unwired: 1 in, 2 out]
        n501 = property on="显示：波形图" class="WFGraph (严格)"("YScale.Maximum"=10.0 ("Y标尺.范围:最大值"), "YScale.Minimum"=0.0 ("Y标尺.范围:最大值")) -> ()  [unwired: 2 in, 2 out]
        n502 = local write "变量：原始数据"(w662) -> ()
        n503 = local write "变量：图像缓存数组"(w706) -> ()
        n504 = local write "显示：波形图_预览"(w706) -> ()
        n505 = local write "显示：波形图"(w706) -> ()
        "变量：上次测量时间" <- w660
      }
      event Panel Close; "按钮_退出": Value Change {
        w726 = T3 "" ("状态栏_游标计数")
        n506 = event-data() -> ()  [unwired: 1 in, 3 out]
        n507 = property on="按钮_开始" class="Bool"("DisabledEnum"=T6."Enabled" ("禁用")) -> ()  [unwired: 2 in, 2 out]
        n508 = Initialize Array(nan ("元素"), 8192 ("维数大小")) -> (w737:dbl[])
        n509 = Build Array(w737, w737) -> (w740:dbl[][])
        n510 = local write "变量：图像缓存数组"(w740) -> ()
        n511 = local write "显示：波形图_预览"(w740) -> ()
        n512 = local write "显示：波形图"(w740) -> ()
        n513 = property on="显示：波形图" class="WFGraph (严格)"("Active Cursor"=u32 1 ("活动游标"), "Cursor.Visible"=FALSE ("游标.可见"), "Cursor.Cursor Plot"=1 ("游标.游标关联曲线"), "Cursor.Cursor Name"="" ("游标.游标名")) -> (error out=w718:errorcluster)  [unwired: 2 in, 1 out]
        n514 = property on="按钮_停止" class="Bool (严格)"("DisabledEnum"=T6."Disabled and Grayed Out" ("禁用")) -> ()  [unwired: 2 in, 2 out]
        n515 = property on="显示：波形图" class="WFGraph (严格)"(error in=w718, "Active Cursor"=u32 0 ("活动游标")) -> (error out=w713:errorcluster)  [unwired: 1 in, 1 out]
        n516 = property on="显示：波形图" class="WFGraph (严格)"(error in=w713, "Cursor.Cursor Position"=T5 {"X"=0.0, "Y"=0.0} ("游标.游标位置"), "Cursor.Visible"=FALSE ("游标.可见"), "YScale.Maximum"=10.0 ("Y标尺.范围:最大值"), "YScale.Minimum"=0.0 ("Y标尺.范围:最小值")) -> (error out=w710:errorcluster)  [unwired: 1 in, 1 out]
        n517 = Initialize Array("", 19 ("维数大小")) -> (w731:string[])
        n518 = property on="列表框" class="MCListbox (严格)"() -> ("ItemNames"=w733:string[][])  [unwired: 2 in, 2 out]
        n519 = Replace Array Subset(array=w731, new element="未命名" ("新元素/子数组"), index=0 ("索引")) -> (w722:string[])
        n520 = property on="显示：波形图_预览" class="WFGraph (严格)"(error in=w710, "Cursor.Cursor Position"=T5 {"X"=0.0, "Y"=0.0} ("游标.游标位置"), "Cursor.Visible"=FALSE ("游标.可见")) -> ()  [unwired: 1 in, 2 out]
        n521 = Replace Array Subset(array=w733, new element=w722, index (col)=1 ("禁用的索引 (列)")) -> (w734:string[][])  [unwired: 1 in]
        n522 = property on="列表框" class="MCListbox (严格)"("ItemNames"=w734) -> ()  [unwired: 2 in, 2 out]
        n523 = local write "状态栏_游标状态"(T3 "隐藏" ("状态栏_游标状态")) -> ()
        n524 = local write "状态栏_测量状态"(T3 "停止" ("状态栏_测量状态")) -> ()
        n525 = local write "状态栏_游标计数"(w726) -> ()
        n526 = local write "状态栏_游标道址"(w726) -> ()
        n527 = local write "状态栏_计数率"(T3 "" ("状态栏_计数率")) -> ()
      }
      event "按钮_开始": Value Change {
        n528 = event-data() -> ()  [unwired: 1 in, 1 out]
        n529 = local read "变量：剩余使用时间"() -> (w744:dbl)
        n530 = local read "状态：停止变量"() -> (w746:bool)
        n531 = Greater?(x=w744, y=0.0) -> (0:w742:bool)
        n532 = And(x=w746, y=w742) -> (x .and. y?=w745:bool)
        n533 = case shown="真" w745 {
          frame False {
          }
          frame True {
            n534 = stacked-sequence {
              frame #0 {
                w756 = ""
                w770 = T6."Disabled and Grayed Out" ("禁用")
                n535 = local read "状态：本次测量和上次未完成测量时间和"() -> (w747:dbl)
                n536 = local read "变量：每次测量计划用时"() -> (w749:u16)
                n537 = local write "状态：停止变量"(FALSE ("停止变量")) -> ()
                n538 = local read "设置：信号极性（正T）"() -> (w750:bool)
                n539 = local read "设置：甄别后阈值"() -> (w752:u16)
                n540 = local read "设置：甄别前阈值"() -> (w751:u16)
                n541 = Greater Or Equal?(x=w747, y=w749) -> (x >= y?=w748:bool)
                n542 = case shown="真" w748 {
                  frame False {
                    n543 = local read "状态：本次测试已测时间"() -> (→"状态：上次未完成测试的已测时间":dbl)
                  }
                  frame True {
                    w775 = 0.0 ("状态：上次未完成测试的已测时间")
                    n544 = local read "变量：每次测量计划用时"() -> (w777:u16)
                    n545 = local read "设置：测量时间"() -> (w778:u16)
                    n546 = local write "状态：上次未完成测试的已测时间"(w775) -> ()
                    n547 = local write "状态：本次测量和上次未完成测量时间和"(w775) -> ()
                    n548 = Add(x=w778, y=w777) -> (x+y=w776:u16)
                    n549 = local write "设置：测量时间"(w776) -> ()
                  }
                }
                n550 = call "MCA_init.vi"("下阈值"=w752, "设置：信号极性（正T）"=w750, "上阈值"=w751) -> ()
                n551 = property on="按钮_复位" class="Bool"("DisabledEnum"=T6."Disabled and Grayed Out" ("禁用")) -> ()  [unwired: 2 in, 2 out]
                n552 = property on="按钮_开始" class="Bool"("DisabledEnum"=w770) -> ()  [unwired: 2 in, 2 out]
                n553 = property on="按钮_打开" class="Bool"("DisabledEnum"=w770) -> ()  [unwired: 2 in, 2 out]
                n554 = property on="按钮_保存" class="Bool"("DisabledEnum"=w770) -> ()  [unwired: 2 in, 2 out]
                n555 = property on="按钮_设置" class="Bool"("DisabledEnum"=w770) -> ()  [unwired: 2 in, 2 out]
                n556 = local read "显示：列表显示内容"() -> (w757:string[])
                n557 = Get Date/Time In Seconds() -> (seconds since 1Jan1904=w755:timestamp)
                n558 = Get Date/Time String(date format (0)=enum16{"short", "long", "abbreviated"}."long" ("日期格式(0)"), seconds (now)=w755) -> (date string=w753:string)  [unwired: 1 in, 1 out]
                n559 = property on="按钮_停止" class="Bool (严格)"("DisabledEnum"=T6."Enabled" ("禁用")) -> ()  [unwired: 2 in, 2 out]
                n560 = Replace Array Subset(array=w757, new element #1=w753, index #1=7 ("索引"), new element #2=w756, index #2=8 ("索引"), new element #3=w756, index #3=17 ("索引"), new element #4=w756, index #4=12 ("索引"), new element #5=w756, index #5=13 ("索引"), new element #6=w756, index #6=14 ("索引"), new element #7=w756, index #7=15 ("索引"), new element #8=w756, index #8=16 ("索引")) -> (w759:string[])
                n561 = local write "显示：列表显示内容"(w759) -> ()
                n562 = local write "状态栏_计数率"(T3 "" ("状态栏_计数率")) -> ()
                n563 = local write "状态栏_测量状态"(T3 "正在测量..." ("状态栏_测量状态")) -> ()
                "状态：刷新次数" <- 1
              }
              frame #1 {
                n564 = Tick Count (ms)() -> (millisecond timer value=w779:u32)
                "状态：测量开始时间" <- w779
                n565 = while {
                  tunnel: w779 -> [w781]
                  stop <- w782 stop-if-true
                  n566 = stacked-sequence {
                    tunnel: w781 -> [w786 _ _]
                    frame #0 {
                      n567 = while {
                        tunnel: w786 -> [w797]
                        stop <- w803 stop-if-true
                        n568 = local read "状态：刷新次数"() -> (w810:i32)
                        n569 = local read "设置：刷新频率"() -> (w809:u16)
                        n570 = local read "变量：上次测量时间"() -> (w790:dbl)
                        n571 = Tick Count (ms)() -> (millisecond timer value=w798:u32)
                        n572 = call "MCA_count.vi"() -> ("多道计数"=w787:i32)
                        "变量：实时计数" <- w787
                        n573 = Subtract(x=w798, y=w797) -> (x-y=w800:u32)
                        n574 = Multiply(x=w810, y=w809) -> (x*y=w808:i32)
                        n575 = Divide(x=w800, y=u32 1000) -> (x/y=w788:dbl)
                        n576 = Greater Or Equal?(x=w787, y=w808) -> (x >= y?=w807:bool)
                        n577 = Add(x=w790, y=w788) -> (x+y=w789:dbl)
                        n578 = local read "变量：每次测量计划用时"() -> (w804:u16)
                        n579 = local read "状态：停止变量"() -> (w805:bool)
                        n580 = case shown="真" w807 {
                          tunnel: [FALSE TRUE] -> w806
                          frame False {
                          }
                          frame True {
                            n581 = local read "状态：刷新次数"() -> (w814:i32)
                            n582 = Increment(x=w814) -> (x+1=w813:i32)
                            n583 = local write "状态：刷新次数"(w813) -> ()
                          }
                        }
                        n584 = local read "显示：列表显示内容"() -> (w795:string[])
                        n585 = Number To Decimal String(number=w789) -> (decimal integer string=w793:string)  [unwired: 1 in]
                        n586 = Concatenate Strings(w793, "秒" ("字符串")) -> (w791:string)
                        n587 = Greater Or Equal?(x=w788, y=w804) -> (x >= y?=w801:bool)
                        n588 = Or(x=w806, y=w805) -> (x .or. y?=w802:bool)
                        n589 = Replace Array Subset(array=w795, new element=w791, index=8 ("索引")) -> (w796:string[])
                        n590 = Or(x=w802, y=w801) -> (x .or. y?=w803:bool)
                        n591 = local write "显示：列表显示内容"(w796) -> ()
                      }
                    }
                    frame #1 {
                      # "冗余是为了保证先计算实时计数率，再赋给下次计算的初始值"
                      n592 = local read "变量：实时计数"() -> (w824:i32)
                      n593 = local read "状态：测量开始时间"() -> (w836:u32)
                      n594 = local read "变量 ： 上次测量总计数"() -> (w842:u32)
                      n595 = local read "变量：上次测量时间"() -> (w840:dbl)
                      n596 = Tick Count (ms)() -> (millisecond timer value=w833:u32)
                      n597 = local read "变量 : 实时总计数"() -> (w851:u64)
                      n598 = local read "状态：已测时间"() -> (w843:dbl)
                      n599 = Subtract(x=w833, y=w836) -> (x-y=w835:u32)
                      n600 = Divide(x=w835, y=u32 1000) -> (x/y=w815:dbl)
                      "状态：本次测试已测时间" <- w815
                      n601 = Add(x=w824, y=w842) -> (x+y=w841:u32)
                      n602 = Subtract(x=w824, y=w851) -> (x-y=w849:u64)
                      n603 = local read "状态：上次未完成测试的已测时间"() -> (w817:dbl)
                      n604 = Subtract(x=w815, y=w843) -> (x-y=w847:dbl)
                      n605 = Divide(x=w849, y=w847) -> (x/y=w844:dbl)
                      n606 = Number To Decimal String(number=w844) -> (decimal integer string=w845:string)  [unwired: 1 in]
                      n607 = Add(x=w840, y=w815) -> (x+y=w823:dbl)
                      n608 = local read "状态：已测时间"() -> (w846:dbl)
                      n609 = Add(x=w849, y=w851) -> (x+y=w850:u64)
                      n610 = local write "状态栏_计数率"(w845) -> ()
                      n611 = local write "变量 : 实时总计数"(w850) -> ()
                      n612 = Add(x=w846, y=w847) -> (x+y=w848:dbl)
                      n613 = local write "状态：已测时间"(w848) -> ()
                      n614 = Add(x=w817, y=w815) -> (x+y=→"状态：本次测量和上次未完成测量时间和":dbl)
                      n615 = local read "设置：测量时间"() -> (w818:u16)
                      n616 = Number To Decimal String(number=w841) -> (decimal integer string=w832:string)  [unwired: 1 in]
                      n617 = Divide(x=w841, y=w823) -> (x/y=w838:dbl)
                      n618 = Number To Decimal String(number=w823) -> (decimal integer string=w828:string)  [unwired: 1 in]
                      n619 = Number To Decimal String(number=w838) -> (decimal integer string=w839:string)  [unwired: 1 in]
                      n620 = Number To Decimal String(number=w818) -> (decimal integer string=w822:string)  [unwired: 1 in]
                      n621 = local read "显示：列表显示内容"() -> (w826:string[])
                      n622 = Concatenate Strings(w828, "秒" ("字符串")) -> (w827:string)
                      n623 = Concatenate Strings(w822, "秒" ("字符串")) -> (w819:string)
                      n624 = Replace Array Subset(array=w826, new element #1=w827, index #1=8 ("索引"), new element #2=w832, index #2=10 ("索引"), new element #3=w839, index #3=11 ("索引"), new element #4=w819, index #4=1 ("索引")) -> (w830:string[])
                      n625 = local write "显示：列表显示内容"(w830) -> ()
                    }
                    frame #2 {
                      n626 = local read "变量：上次测量原始数据"() -> (w867:dbl[])
                      n627 = local read "MCA道宽修正数组"() -> (w854:ext[])
                      n628 = local read "设置：幅度谱总道数"() -> (w866:u32)
                      n629 = call "MCA_slave.vi"() -> ("波形图"=w852:i32[])
                      n630 = for {
                        tunnel: w852 -> [w921] mode=indexing
                        tunnel: w867 -> [w922] mode=indexing
                        tunnel: w854 -> [w919] mode=indexing
                        tunnel: [w916] -> w853 mode=indexing
                        n631 = Add(x=w921, y=w922) -> (x+y=w920:dbl)
                        n632 = Multiply(x=w920, y=w919) -> (x*y=w918:ext)
                        n633 = Round To Nearest(number=w918) -> (nearest integer value=w917:ext)
                        n634 = To Unsigned Long Integer(number=w917) -> (unsigned 32bit integer=w916:u32)
                      }
                      n635 = Divide(x=8192.0, y=w866) -> (x/y=w864:dbl)
                      n636 = case shown="8" w864 {
                        tunnel: [w877 w879 w888 w903] -> w855
                        tunnel: w853 -> [w877 w878 w885 w896]
                        frame 1, Default {
                        }
                        frame 2 {
                          n637 = Decimate 1D Array(w878) -> (w880:u32[], w881:u32[])
                          n638 = for {
                            tunnel: w881 -> [w883] mode=indexing
                            tunnel: w880 -> [w884] mode=indexing
                            tunnel: [w882] -> w879 mode=indexing
                            n639 = Add(x=w884, y=w883) -> (x+y=w882:u32)
                          }
                        }
                        frame 4 {
                          n640 = Decimate 1D Array(w885) -> (w889:u32[], w890:u32[], w887:u32[], w886:u32[])
                          n641 = for {
                            tunnel: w890 -> [w894] mode=indexing
                            tunnel: w889 -> [w895] mode=indexing
                            tunnel: [w893] -> w888 mode=indexing
                            tunnel: w887 -> [w892] mode=indexing
                            tunnel: w886 -> [w891] mode=indexing
                            n642 = Compound Arithmetic op=ADD(w895, w894, w892, w891) -> (w893:u32)
                          }
                        }
                        frame 8 {
                          n643 = Decimate 1D Array(w896) -> (w904:u32[], w905:u32[], w902:u32[], w901:u32[], w900:u32[], w899:u32[], w898:u32[], w897:u32[])
                          n644 = for {
                            tunnel: w905 -> [w913] mode=indexing
                            tunnel: w904 -> [w914] mode=indexing
                            tunnel: [w912] -> w903 mode=indexing
                            tunnel: w902 -> [w911] mode=indexing
                            tunnel: w901 -> [w910] mode=indexing
                            tunnel: w900 -> [w909] mode=indexing
                            tunnel: w899 -> [w908] mode=indexing
                            tunnel: w898 -> [w907] mode=indexing
                            tunnel: w897 -> [w906] mode=indexing
                            n645 = Compound Arithmetic op=ADD(w914, w913, w911, w910, w909, w908, w907, w906) -> (w912:u32)
                          }
                        }
                      }
                      n646 = local write "变量：原始数据"(w852) -> ()
                      n647 = local read "变量：感兴区终点道址"() -> (w868:dbl)
                      n648 = local read "变量：感兴区起点道址"() -> (w869:dbl)
                      n649 = for {
                        tunnel: [nan] -> w874 mode=indexing
                        tunnel: w855 -> [_] mode=indexing
                      }
                      n650 = Array Max & Min(array=w855) -> (max value=w859:u32)  [unwired: 3 out]
                      n651 = Multiply(x=w859, y=1.1) -> (x*y=w860:dbl)
                      n652 = Build Array(w855, w874) -> (w870:dbl[][])
                      n653 = local write "变量：图像缓存数组"(w870) -> ()
                      n654 = Index Array(array=w870, index (row)=0 ("索引 (行)")) -> (element=w873:dbl[])  [unwired: 1 in]
                      n655 = Less?(x=w860, y=10.0) -> (x < y?=w861:bool)
                      n656 = case shown="真" w861 {
                        tunnel: w860 -> [w875 _]
                        tunnel: [w875 10.0] -> w856
                        frame False {
                        }
                        frame True {
                        }
                      }
                      n657 = call "一线双色计算.vi"("输入一维数组"=w873, "right corsor"=w868, "left corsor"=w869) -> ("输出波形数组"=w872:dbl[][])
                      n658 = local write "显示：波形图_预览"(w872) -> ()
                      n659 = property on="显示：波形图" class="WFGraph (严格)"("YScale.Maximum"=w856, "YScale.Minimum"=0.0 ("Y标尺.范围:最小值")) -> ()  [unwired: 2 in, 2 out]
                      n660 = property on="显示：波形图_预览" class="WFGraph (严格)"("YScale.Maximum"=w856, "YScale.Minimum"=0.0 ("Y标尺.范围:最小值")) -> ()  [unwired: 2 in, 2 out]
                      n661 = local write "显示：波形图"(w872) -> ()
                    }
                  }
                  n662 = local read "状态：本次测量和上次未完成测量时间和"() -> (w780:dbl)
                  n663 = local read "变量：每次测量计划用时"() -> (w785:u16)
                  n664 = local read "状态：停止变量"() -> (w783:bool)
                  n665 = Greater Or Equal?(x=w780, y=w785) -> (x >= y?=w784:bool)
                  n666 = Or(x=w784, y=w783) -> (x .or. y?=w782:bool)
                }
              }
              frame #2 {
                n667 = flat-sequence {
                  frame #0 {
                    n668 = local write "状态：停止变量"(TRUE ("停止变量")) -> ()
                    n669 = Wait (ms)(milliseconds to wait=u32 100 ("等待时间（毫秒）")) -> ()  [unwired: 1 out]
                  }
                  frame #1 {
                    w950 = T6."Enabled" ("禁用")
                    n670 = local read "变量：上次测量原始数据"() -> (w949:dbl[])
                    n671 = call "MCA_main_read.vi"() -> ("波形图"=w925:i32[])
                    n672 = local read "MCA道宽修正数组"() -> (w932:ext[])
                    n673 = local read "设置：幅度谱总道数"() -> (w948:u32)
                    n674 = local write "状态栏_测量状态"(T3 "停止" ("状态栏_测量状态")) -> ()
                    n675 = local write "状态栏_计数率"(T3 "" ("状态栏_计数率")) -> ()
                    n676 = local write "变量：原始数据"(w925) -> ()
                    n677 = for {
                      tunnel: w925 -> [w1021] mode=indexing
                      tunnel: w949 -> [w1022] mode=indexing
                      tunnel: [w1020] -> w930 mode=indexing
                      n678 = Add(x=w1021, y=w1022) -> (x+y=w1020:dbl)
                    }
                    n679 = Divide(x=8192.0, y=w948) -> (x/y=w946:dbl)
                    n680 = for {
                      tunnel: w932 -> [w978] mode=indexing
                      tunnel: w930 -> [w979] mode=indexing
                      tunnel: [w975] -> w931 mode=indexing
                      n681 = Multiply(x=w979, y=w978) -> (x*y=w977:ext)
                      n682 = Round To Nearest(number=w977) -> (nearest integer value=w976:ext)
                      n683 = To Unsigned Long Integer(number=w976) -> (unsigned 32bit integer=w975:u32)
                    }
                    n684 = local write "变量：上次测量原始数据"(w930) -> ()
                    n685 = case shown="1, 默认" w946 {
                      tunnel: w931 -> [w982 w986 w995 w1010]
                      tunnel: [w982 w983 w992 w1007] -> w939
                      frame 1, Default {
                      }
                      frame 2 {
                        n686 = Decimate 1D Array(w986) -> (w984:u32[], w985:u32[])
                        n687 = for {
                          tunnel: w985 -> [w988] mode=indexing
                          tunnel: w984 -> [w989] mode=indexing
                          tunnel: [w987] -> w983 mode=indexing
                          n688 = Add(x=w989, y=w988) -> (x+y=w987:u32)
                        }
                      }
                      frame 4 {
                        n689 = Decimate 1D Array(w995) -> (w993:u32[], w994:u32[], w991:u32[], w990:u32[])
                        n690 = for {
                          tunnel: w994 -> [w999] mode=indexing
                          tunnel: w993 -> [w1000] mode=indexing
                          tunnel: [w998] -> w992 mode=indexing
                          tunnel: w991 -> [w997] mode=indexing
                          tunnel: w990 -> [w996] mode=indexing
                          n691 = Compound Arithmetic op=ADD(w1000, w999, w997, w996) -> (w998:u32)
                        }
                      }
                      frame 8 {
                        n692 = Decimate 1D Array(w1010) -> (w1008:u32[], w1009:u32[], w1006:u32[], w1005:u32[], w1004:u32[], w1003:u32[], w1002:u32[], w1001:u32[])
                        n693 = for {
                          tunnel: w1009 -> [w1018] mode=indexing
                          tunnel: w1008 -> [w1019] mode=indexing
                          tunnel: [w1017] -> w1007 mode=indexing
                          tunnel: w1006 -> [w1016] mode=indexing
                          tunnel: w1005 -> [w1015] mode=indexing
                          tunnel: w1004 -> [w1014] mode=indexing
                          tunnel: w1003 -> [w1013] mode=indexing
                          tunnel: w1002 -> [w1012] mode=indexing
                          tunnel: w1001 -> [w1011] mode=indexing
                          n694 = Compound Arithmetic op=ADD(w1019, w1018, w1016, w1015, w1014, w1013, w1012, w1011) -> (w1017:u32)
                        }
                      }
                    }
                    n695 = property on="按钮_开始" class="Bool"("DisabledEnum"=w950) -> ()  [unwired: 2 in, 2 out]
                    n696 = property on="按钮_复位" class="Bool"("DisabledEnum"=w950) -> ()  [unwired: 2 in, 2 out]
                    n697 = property on="按钮_保存" class="Bool"("DisabledEnum"=w950) -> ()  [unwired: 2 in, 2 out]
                    n698 = property on="按钮_设置" class="Bool"("DisabledEnum"=w950) -> ()  [unwired: 2 in, 2 out]
                    n699 = property on="按钮_打开" class="Bool"("DisabledEnum"=w950) -> ()  [unwired: 2 in, 2 out]
                    n700 = property on="按钮_停止" class="Bool (严格)"("DisabledEnum"=T6."Disabled and Grayed Out" ("禁用")) -> ()  [unwired: 2 in, 2 out]
                    n701 = local read "变量：上次测量时间"() -> (w927:dbl)
                    n702 = local read "状态：已测时间"() -> (w928:dbl)
                    n703 = for {
                      tunnel: w939 -> [_] mode=indexing
                      tunnel: [nan] -> w974 mode=indexing
                    }
                    n704 = local read "变量：感兴区起点道址"() -> (w954:dbl)
                    n705 = local read "变量：感兴区终点道址"() -> (w955:dbl)
                    n706 = Array Max & Min(array=w939) -> (max value=w940:u32)  [unwired: 3 out]
                    n707 = Add(x=w928, y=w927) -> (x+y=w926:dbl)
                    n708 = Build Array(w939, w974) -> (w959:dbl[][])
                    n709 = local write "变量：图像缓存数组"(w959) -> ()
                    n710 = local write "变量：上次测量时间"(w926) -> ()
                    n711 = Multiply(x=w940, y=1.1) -> (x*y=w941:dbl)
                    n712 = Index Array(array=w959, index (row)=0 ("索引 (行)")) -> (element=w956:dbl[])  [unwired: 1 in]
                    n713 = Less?(x=w941, y=10.0) -> (x < y?=w942:bool)
                    n714 = call "一线双色计算.vi"("输入一维数组"=w956, "right corsor"=w955, "left corsor"=w954) -> ("输出波形数组"=w957:dbl[][])
                    n715 = case shown="假" w942 {
                      tunnel: w941 -> [w980 _]
                      tunnel: [w980 10.0] -> w936
                      frame False {
                      }
                      frame True {
                      }
                    }
                    n716 = Add Array Elements(numeric array=w939) -> (sum=w945:u32)
                    n717 = Round To Nearest(number=w926) -> (nearest integer value=w929:dbl)
                    n718 = local write "显示：波形图"(w957) -> ()
                    n719 = local write "显示：波形图_预览"(w957) -> ()
                    n720 = Number To Decimal String(number=w926) -> (decimal integer string=w953:string)  [unwired: 1 in]
                    n721 = local read "显示：列表显示内容"() -> (w972:string[])
                    n722 = Divide(x=w945, y=w929) -> (x/y=w961:dbl)
                    n723 = local write "变量 ： 上次测量总计数"(w945) -> ()
                    n724 = Get Date/Time String(date format (0)=enum16{"short", "long", "abbreviated"}."long" ("日期格式(0)"), want seconds? (F)=TRUE ("需要秒？(F)")) -> (date string=w965:string, time string=w964:string)  [unwired: 1 in]
                    n725 = Number To Decimal String(number=w961) -> (decimal integer string=w960:string)  [unwired: 1 in]
                    n726 = Number To Decimal String(number=w945) -> (decimal integer string=w967:string)  [unwired: 1 in]
                    n727 = Concatenate Strings(w953, "秒" ("字符串")) -> (w933:string)
                    n728 = property on="显示：波形图" class="WFGraph (严格)"("YScale.Maximum"=w936, "YScale.Minimum"=0.0 ("Y标尺.范围:最小值")) -> ()  [unwired: 2 in, 2 out]
                    n729 = property on="显示：波形图_预览" class="WFGraph (严格)"("YScale.Maximum"=w936, "YScale.Minimum"=0.0 ("Y标尺.范围:最小值")) -> ()  [unwired: 2 in, 2 out]
                    n730 = Replace Array Subset(array=w972, new element #1=w965, index #1=7 ("索引"), new element #2=w964, index #2=9 ("索引"), new element #3=w967, index #3=10 ("索引"), new element #4=w960, index #4=11 ("索引"), new element #5=w933, index #5=8 ("索引")) -> (w971:string[])
                    n731 = local write "显示：列表显示内容"(w971) -> ()
                  }
                }
              }
              frame #3 {
                n732 = Get Date/Time In Seconds() -> (seconds since 1Jan1904=w1039:timestamp)
                n733 = Get Date/Time String(date format (0)=enum16{"short", "long", "abbreviated"}."long" ("日期格式(0)"), seconds (now)=w1039, want seconds? (F)=TRUE ("需要秒？(F)")) -> (date string=w1040:string, time string=w1029:string)
                n734 = Replace Substring(2:1 ("长度（子字符串长度）"), 3:2 ("偏移量(0)"), 4:"时" ("子字符串(\"\")"), 5:w1029) -> (1:w1027:string)  [unwired: 1 out]
                n735 = Current VI's Path() -> (path=w1052:path)
                n736 = Strip Path(path=w1052) -> (stripped path=w1045:path)  [unwired: 1 out]
                n737 = Replace Substring(2:1 ("长度（子字符串长度）"), 3:6 ("偏移量(0)"), 4:"分" ("子字符串(\"\")"), 5:w1027) -> (1:w1026:string)  [unwired: 1 out]
                n738 = Build Path(base path=w1045, name or relative path="data") -> (appended path=w1043:path)
                n739 = local read "显示：列表显示内容"() -> (w1051:string[])
                n740 = Replace Substring(2:1 ("长度（子字符串长度）"), 3:10 ("偏移量(0)"), 4:"秒" ("子字符串(\"\")"), 5:w1026) -> (1:w1028:string)  [unwired: 1 out]
                n741 = Concatenate Strings(w1040, w1028) -> (w1025:string)
                n742 = Build Path(base path=w1043, name or relative path=w1025) -> (appended path=w1042:path)
                n743 = Index Array(array=w1051, index #1=5 ("索引"), index #2=6 ("索引")) -> (element #1=w1048:string, element #2=w1047:string)
                n744 = property on="列表框" class="MCListbox (严格)"() -> ("ItemNames"=w1065:string[][])  [unwired: 2 in, 2 out]
                n745 = Concatenate Strings(w1048, w1047) -> (w1046:string)
                n746 = TDMS Open(5:FALSE ("创建索引文件？(T)"), 10:T7."create or replace" ("操作(0:open)"), 11:w1042) -> (0:w1057:errorcluster, 3:w1067:refnum<k34>)  [unwired: 4 in]
                n747 = Index Array(array=w1065, index (col)=0 ("禁用的索引 (列)")) -> (element=w1063:string[])  [unwired: 1 in]
                n748 = Replace Array Subset(array=w1051, new element=w1046, index=0 ("索引")) -> (w1062:string[])
                n749 = local write "显示：列表显示内容"(w1062) -> ()
                n750 = Build Array(w1063, w1062) -> (w1054:string[][])
                n751 = TDMS Write(0:w1067, 5:"文件属性" ("组名称输入（无标题）"), 7:string[] ["属性名称", "值"] ("通道名输入（无标题）"), 9:w1054, 11:w1057) -> (4:w1061:refnum<k34>, 15:w1056:errorcluster)  [unwired: 1 in, 2 out]
                n752 = local read "变量：原始数据"() -> (w1053:dbl[])
                n753 = TDMS Write(0:w1061, 5:"数据" ("组名称输入（无标题）"), 7:"计数", 9:w1053, 11:w1056) -> (4:w1058:refnum<k34>, 15:w1055:errorcluster)  [unwired: 1 in, 2 out]
                n754 = TDMS Close(8:w1055, 11:w1058) -> ()  [unwired: 2 out]
              }
            }
          }
        }
      }
    }
  }
  n755 = while {
    stop <- w1073 stop-if-true
    n756 = event shown="[0] 超时" {
      selector: _ -> [_ _]
      dyn-events: _ -> [_ _]
      timeout: 300 -> [_ _]
      tunnel: [_ TRUE] -> w1073
      event Timeout {
        n757 = event-data() -> ()  [unwired: 1 in, 3 out]
        n758 = local read "显示：列表显示内容"() -> (w1082:string[])
        n759 = property on="显示：波形图" class="WFGraph (严格)"("Active Cursor"=u32 0 ("活动游标")) -> (error out=w1080:errorcluster, "Cursor.Visible"=w1079:bool)  [unwired: 2 in, 1 out]
        n760 = property on="列表框" class="MCListbox (严格)"() -> ("ItemNames"=w1094:string[][])  [unwired: 2 in, 2 out]
        n761 = property on="显示：波形图" class="WFGraph (严格)"(error in=w1080) -> (error out=w1077:errorcluster, "Cursor.Cursor X"=w1078:dbl)  [unwired: 1 in, 1 out]
        n762 = Replace Array Subset(array=w1094, new element=w1082, index (col)=1 ("禁用的索引 (列)")) -> (w1095:string[][])  [unwired: 1 in]
        n763 = property on="列表框" class="MCListbox (严格)"("ItemNames"=w1095) -> ()  [unwired: 2 in, 2 out]
        n764 = property on="显示：波形图_预览" class="WFGraph (严格)"(error in=w1077, "Cursor.Cursor X"=w1078) -> ()  [unwired: 1 in, 2 out]
        n765 = case shown="真" w1079 {
          tunnel: w1078 -> [_ w1096]
          tunnel: w1077 -> [_ _]
          frame False {
          }
          frame True {
            n766 = local read "变量：显示数据"() -> (w1099:dbl[])
            n767 = Number To Decimal String(number=w1096) -> (decimal integer string=w1100:string)  [unwired: 1 in]
            n768 = local write "状态栏_游标道址"(w1100) -> ()
            n769 = Index Array(array=w1099, index=w1096) -> (element=w1098:dbl)
            n770 = Number To Decimal String(number=w1098) -> (decimal integer string=w1097:string)  [unwired: 1 in]
            n771 = local write "状态栏_游标计数"(w1097) -> ()
          }
        }
        n772 = UDP Open(11:u16 8080 ("端口")) -> (0:w1075:errorcluster)  [unwired: 4 in, 2 out]
        n773 = Get Date/Time In Seconds() -> (seconds since 1Jan1904=w1092:timestamp)
        n774 = call <vilib>:"Simple Error Handler.vi"("error in (no error)"=w1075) -> ("error?"=w1074:bool)  [unwired: 4 in, 4 out]
        n775 = case shown="假" w1074 {
          tunnel: ["已连接" "未连接"] -> w1083
          frame False {
          }
          frame True {
          }
        }
        n776 = Get Date/Time String(date format (0)=enum16{"short", "long", "abbreviated"}."short" ("日期格式(0)"), seconds (now)=w1092, want seconds? (F)=FALSE ("需要秒？(F)")) -> (date string=w1090:string, time string=w1088:string)
        n777 = Concatenate Strings(w1090, "   " ("字符串"), w1088) -> (→"状态栏_日期":string)
        n778 = Concatenate Strings("核电子学硬件平台" ("字符串"), w1083) -> (→"状态栏_仪器状态":string)
      }
      event "按钮_退出": Value Change; Panel Close {
        n779 = event-data() -> ()  [unwired: 1 in, 3 out]
      }
    }
  }
  n780 = while {
    stop <- FALSE stop-if-true
    n781 = event shown="[1] 前面板关闭" {
      selector: _ -> [_ _]
      dyn-events: _ -> [_ _]
      timeout: _ -> [_ _]
      event Timeout {
        n782 = event-data() -> ()  [unwired: 1 in, 3 out]
      }
      event Panel Close {
        n783 = event-data() -> ()  [unwired: 1 in, 3 out]
        n784 = control-ref of="本VI"() -> (w1105:refnum<vi>)
        n785 = invoke class="VI" method="Abort VI"(reference=w1105) -> ()  [unwired: 2 in, 3 out]
      }
    }
  }
